vi "r3_sensor HDI placingerror.vi"() -> ()   [LabVIEW 2016]
uses:
  Classes/Controllers/Motion/Copy of Motion Folder/Motion.lvclass
  Classes/Controllers/Camera/Copy of Controller Folder/Controller.lvclass
panel:
  out "HDI center position from all time":dbl[][][](array[numeric])
  out "HDI-sensor deviation from all time":dbl[][][](array[numeric])
  out "HDI center position":dbl[][](array[numeric]) format="%#_8g"
  out "HDI bottom right":dbl[][](array[numeric]) format="%#_8g"
  out "HDI bottom left":dbl[][](array[numeric]) format="%#_8g"
  out "HDI top left":dbl[][](array[numeric]) format="%#_8g"
  in  "Default HDI A size":dbl[](array[numeric])=[24.3, 129.2, 78.448, 0.0001904]
  in  "Default HDI B size":dbl[](array[numeric])=[24.3, 101.2, 78.448, 0.0001904]
  in  "default HDI B top letf cross mark":dbl[](array[numeric])=[292.30913, 988.82841, 78.95, 0.00019035373]
  in  "default HDI A top left croos mark":dbl[](array[numeric])=[292.36164, 1091.0109, 78.95, 0.00019104402]
  out "measure times of HDI":dbl
  in  "Default sensor A size":dbl[](array[numeric])=[22.0, 129.5, 78.448, 0.0001904]
  in  "measure HDI position":bool
  in  "south - bottom right":bool
  in  "south - bottom left":bool
  in  "south - upper left":bool
  in  "north - bottom right":bool
  in  "north - bottom left":bool
  in  "north - upper left":bool
  out "HDI - sensor deviation on time":dbl[][](array[numeric]) format="%#_8g"
  out "HDI center position on time":dbl[][](array[numeric]) format="%#_8g"
  in  "default sensor A top left croos mark":dbl[](array[numeric])=[293.11276, 1090.4659, 78.600001, 0.00019004214]
  in  "test":bool
  in  "how much sensors":i32=2
  out "sensor bottom right":dbl[][](array[numeric]) format="%#_8g"
  out "sensor bottom left":dbl[][](array[numeric]) format="%#_8g"
  out "sensor top left":dbl[][](array[numeric]) format="%#_8g"
  out "sensor center position":dbl[][](array[numeric]) format="%#_8g"
  in  "default sensor B top letf cross mark":dbl[](array[numeric])=[293.05065, 988.27536, 78.609997, 0.00018966104]
  in  "Default sensor B size":dbl[](array[numeric])=[22.0, 101.5, 78.448, 0.0001904]
  out "measure times of sensor":dbl
  in  "Parking position":dbl[](array[numeric])=[625.0, 625.0, 0.0, 0.01]
  in  "measure sensor position":bool
  in  "calculate":bool
  in  "go to park":bool
  in  "stop":bool
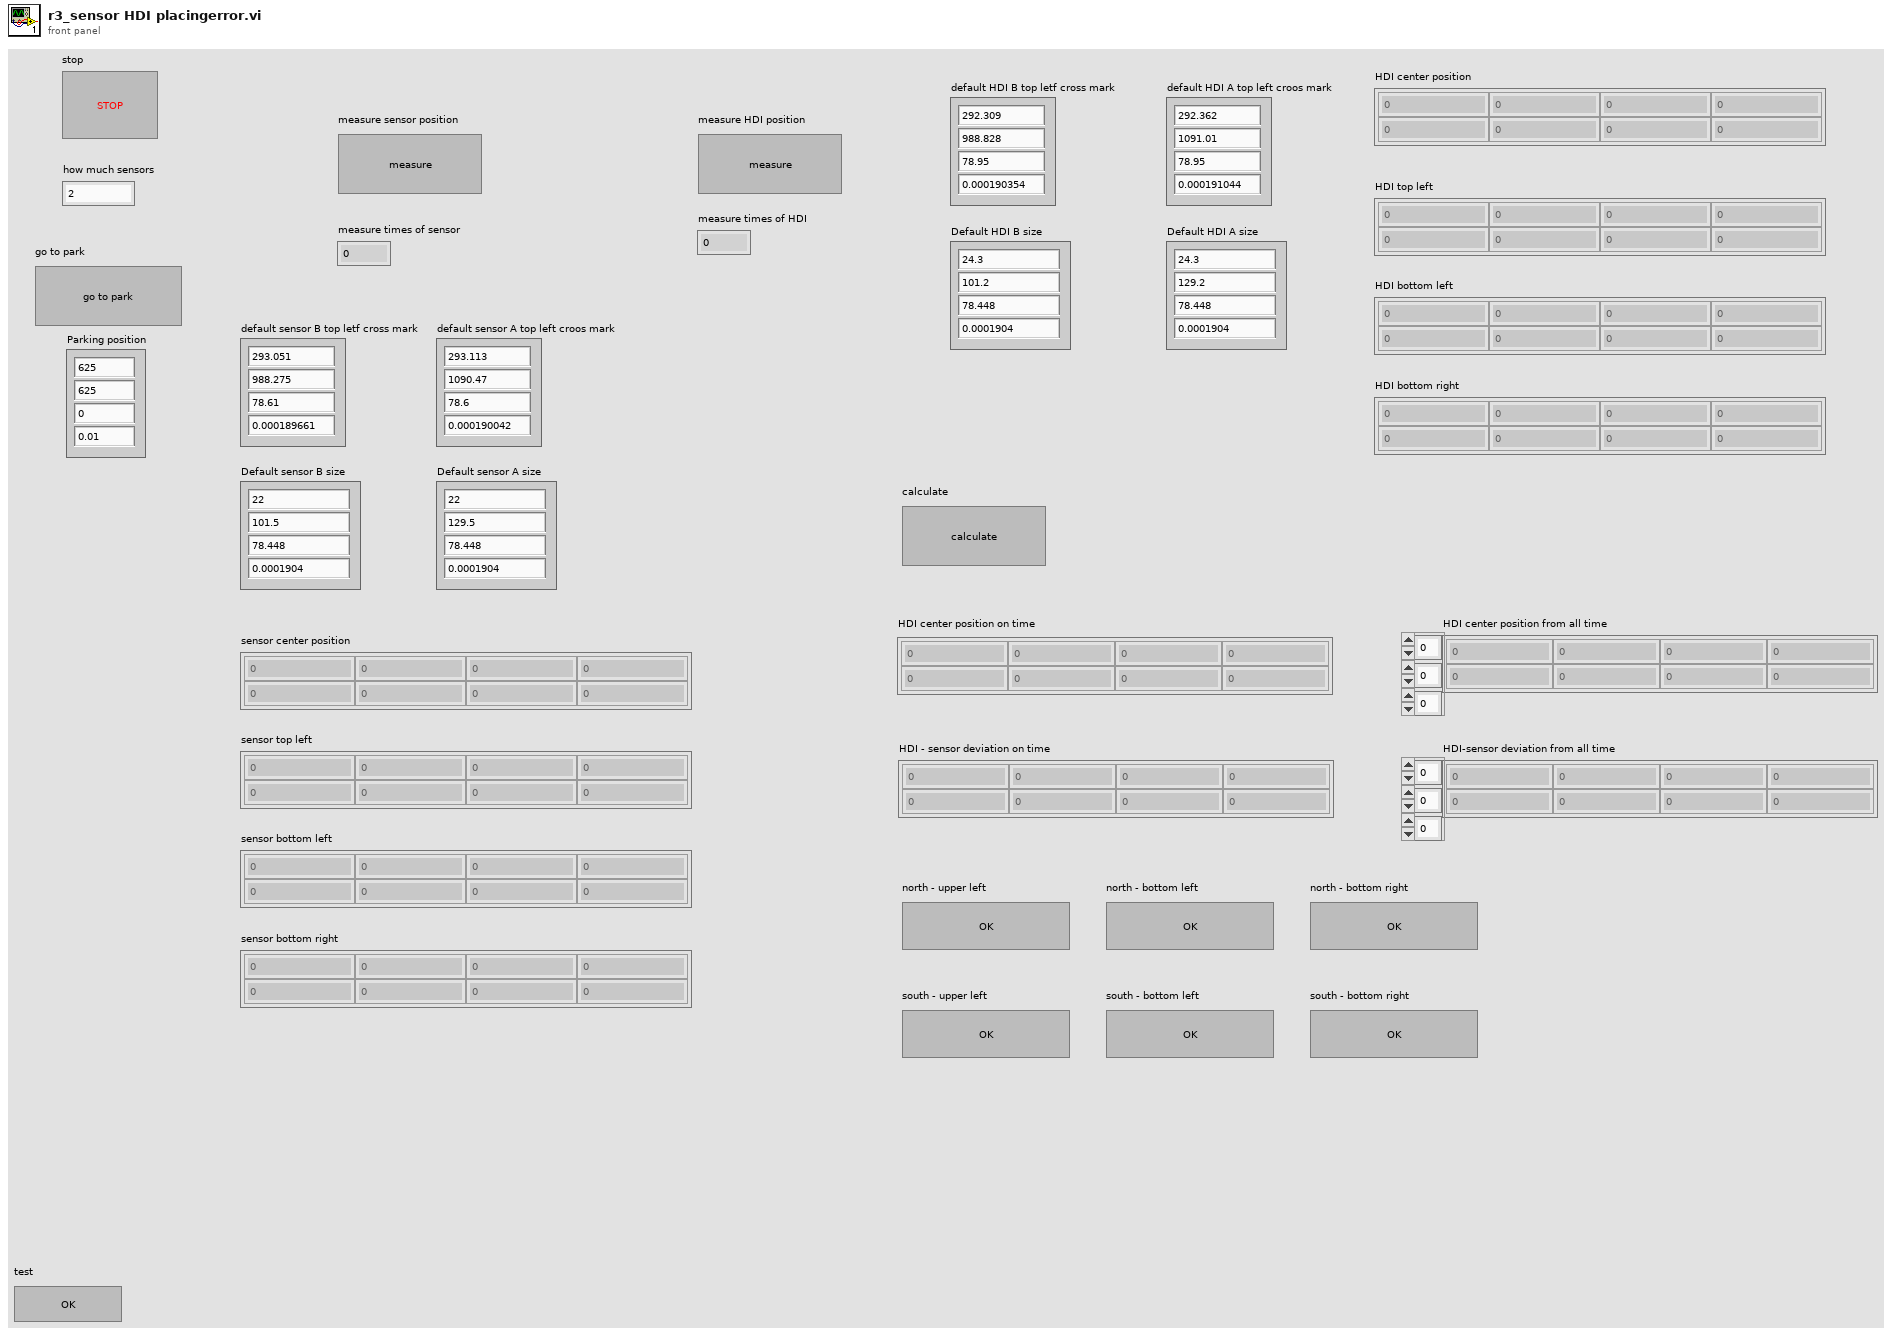
[diagram p1: front panel]
types:
  T1 = typedef "Controller.lvclass/Controllers.ctl" = cluster{"Copy of Motion.lvclass":refnum<class "Motion.lvclass">, "Copy of I-O.lvclass":refnum<class "I-O.lvclass">, "Copy of Dispenser.lvclass":refnum<class "Dispenser.lvclass">}
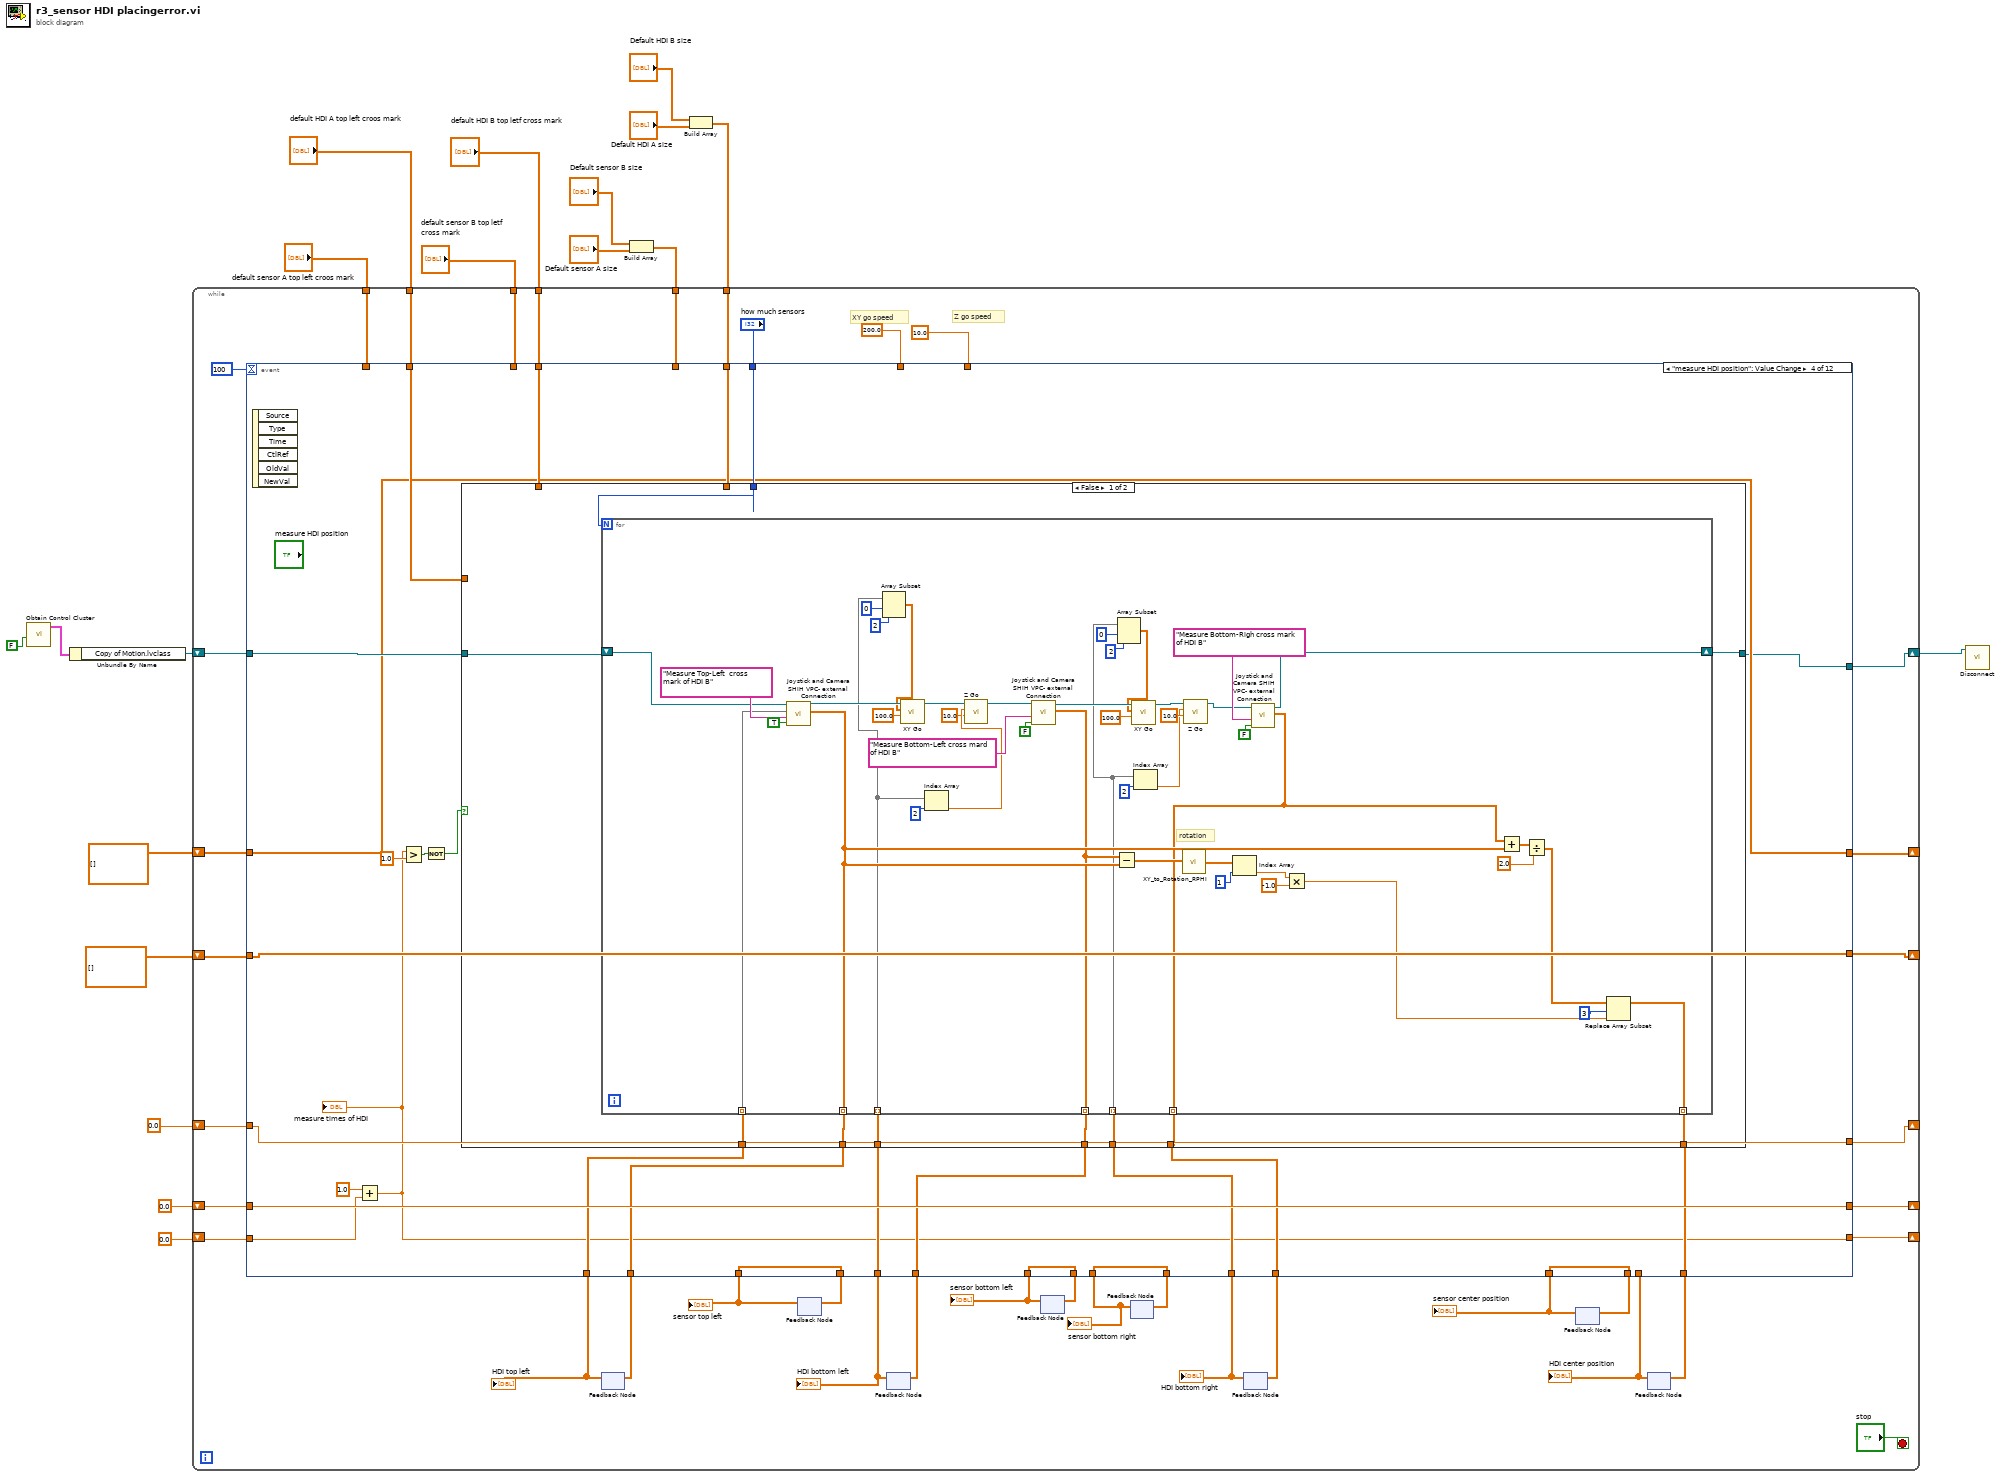
[diagram p0: block diagram]
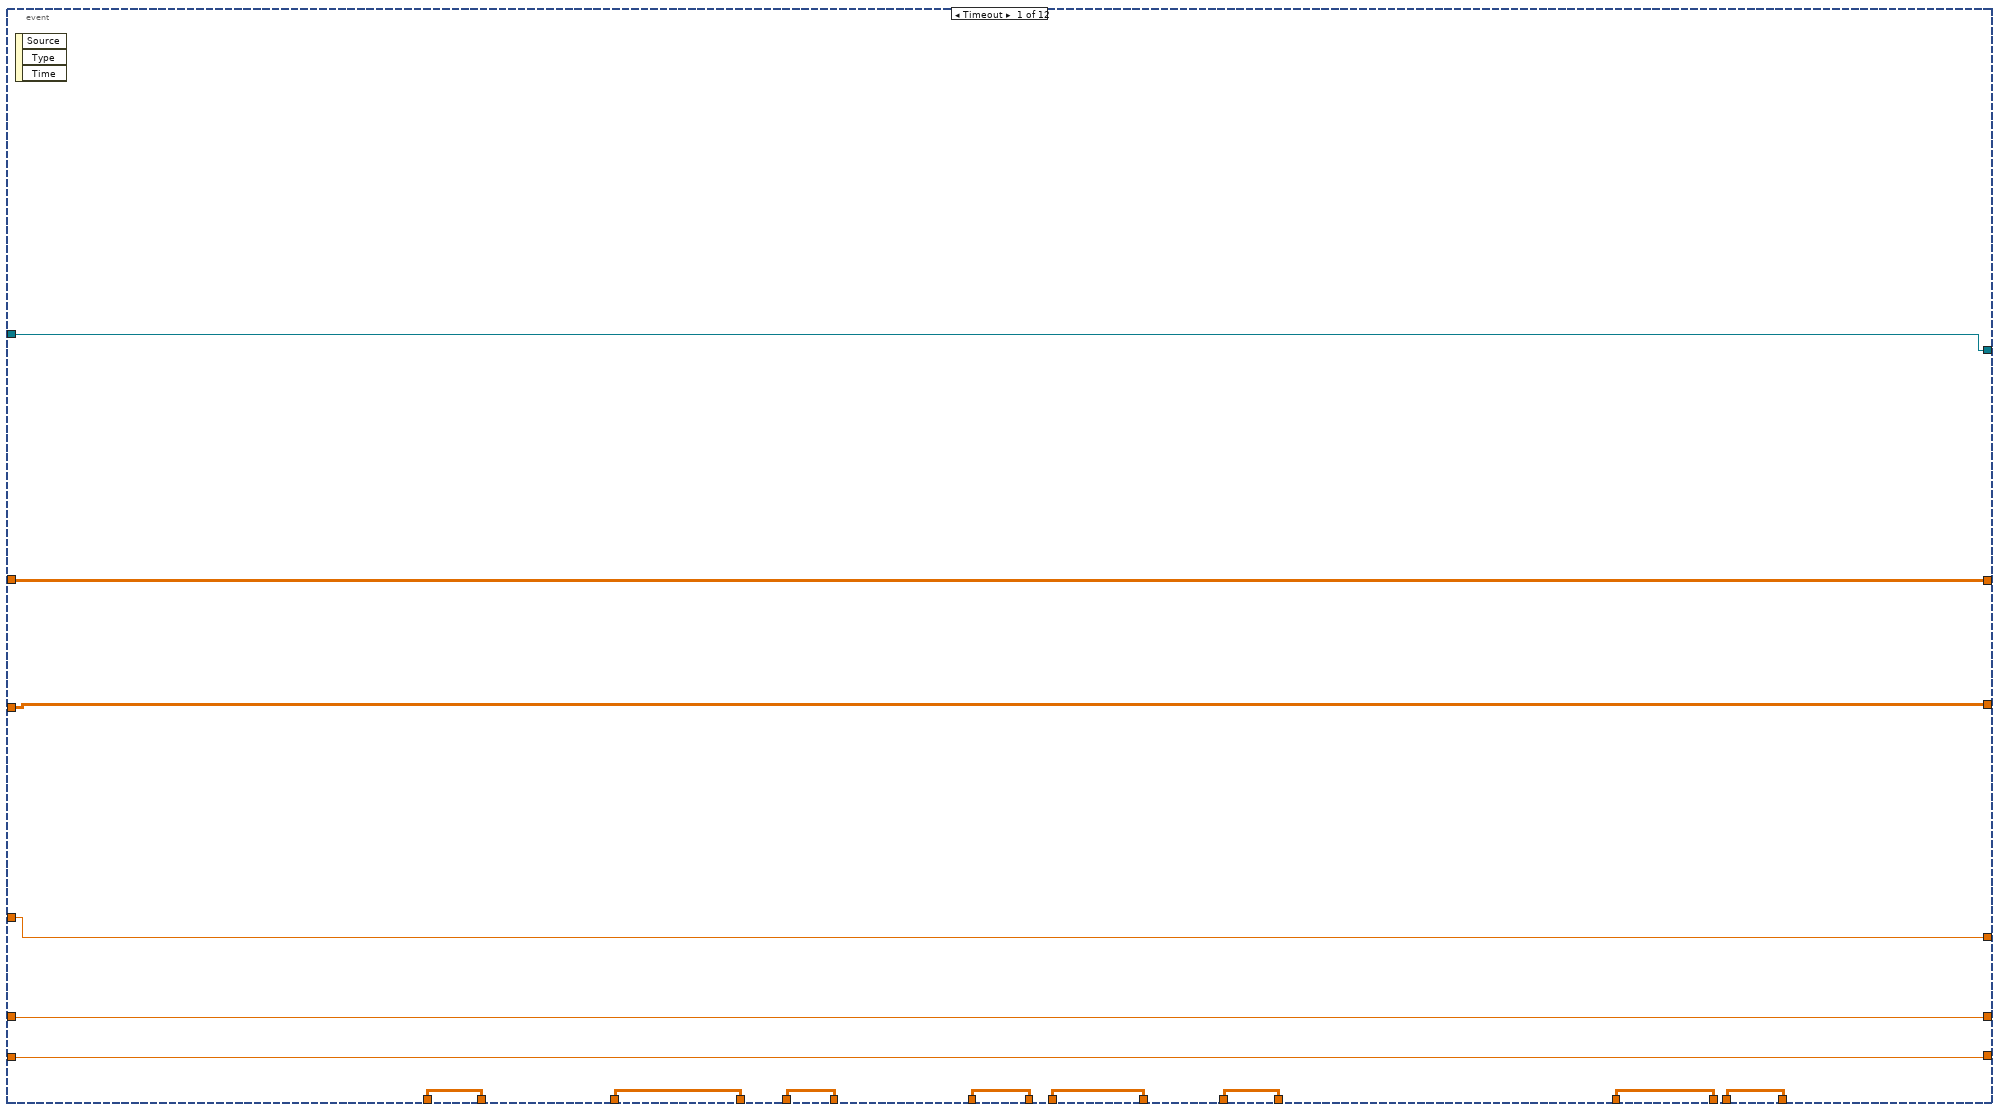
[diagram p2: hidden frame]
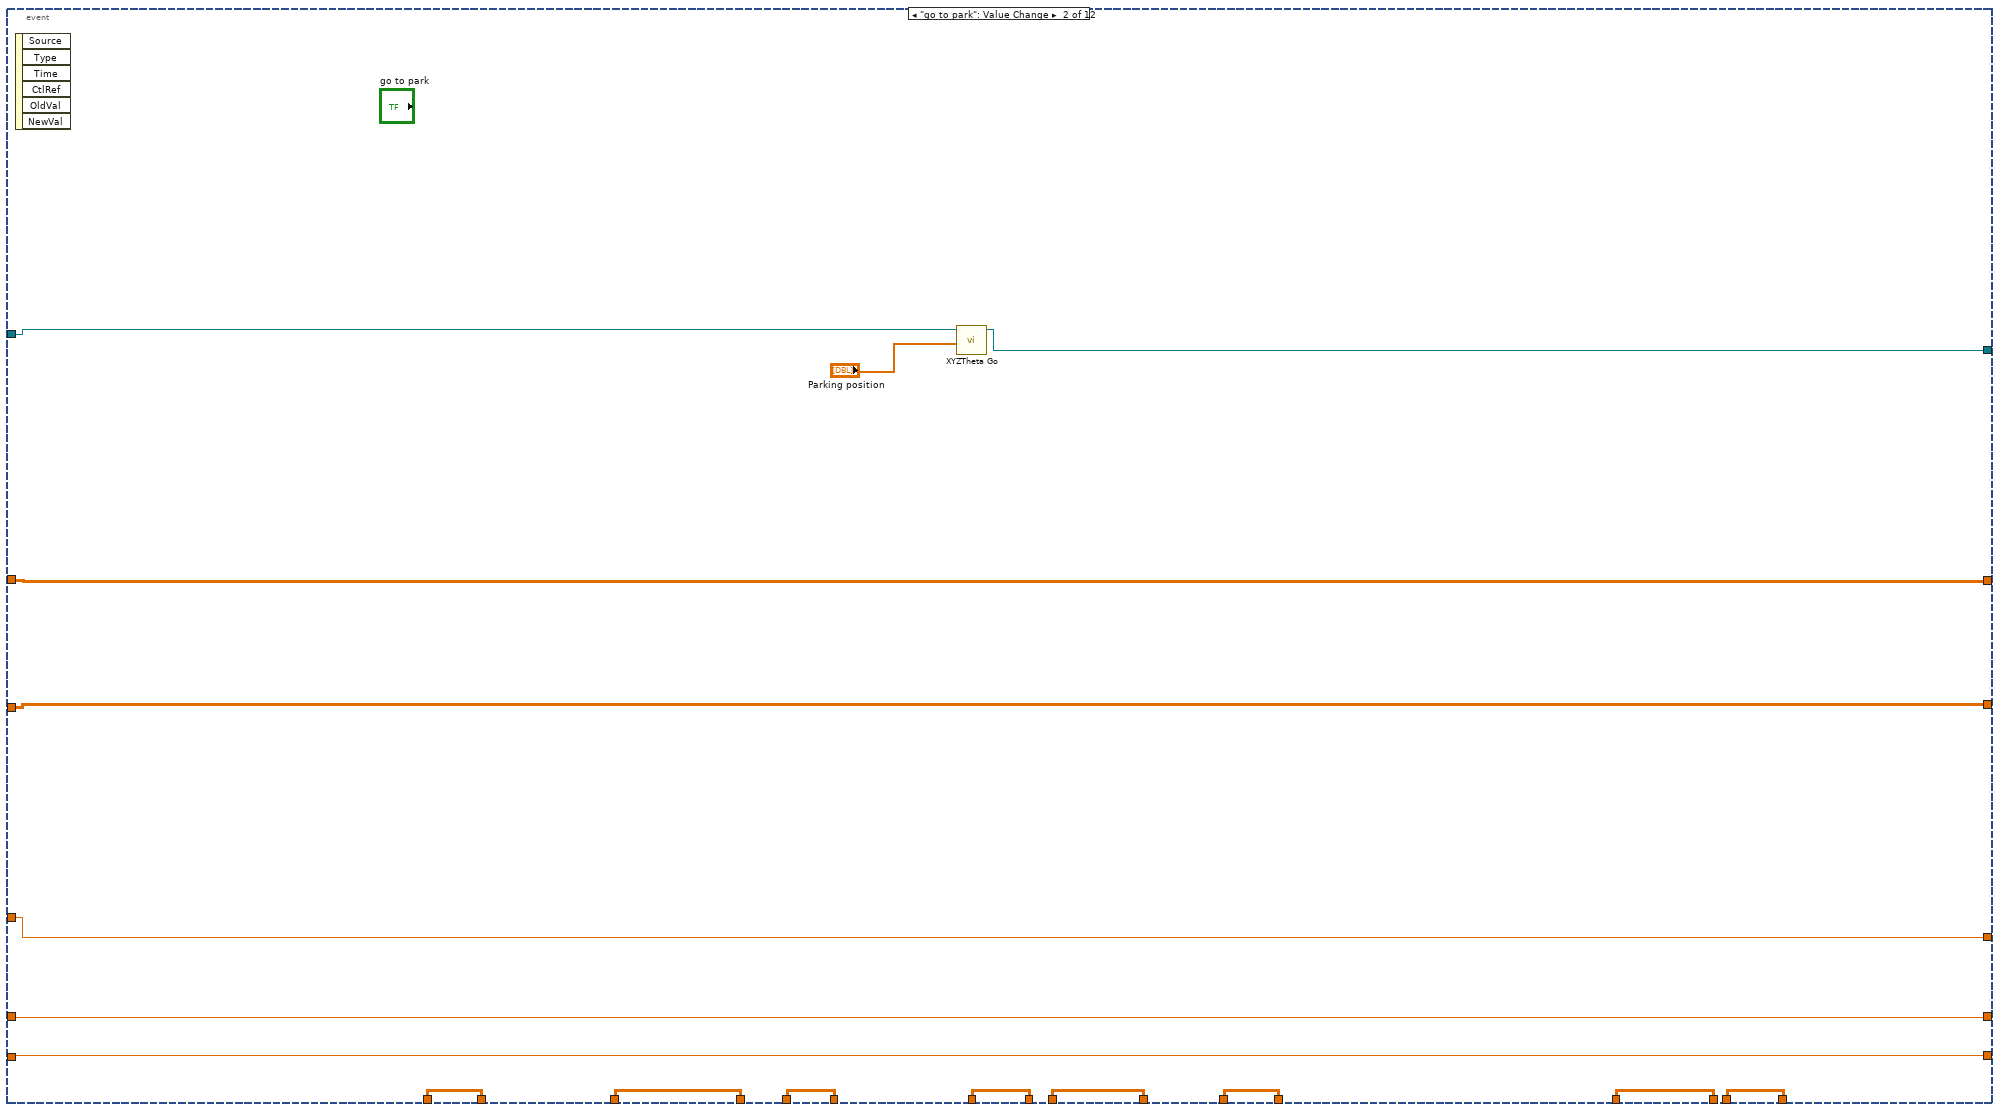
[diagram p3: hidden frame]
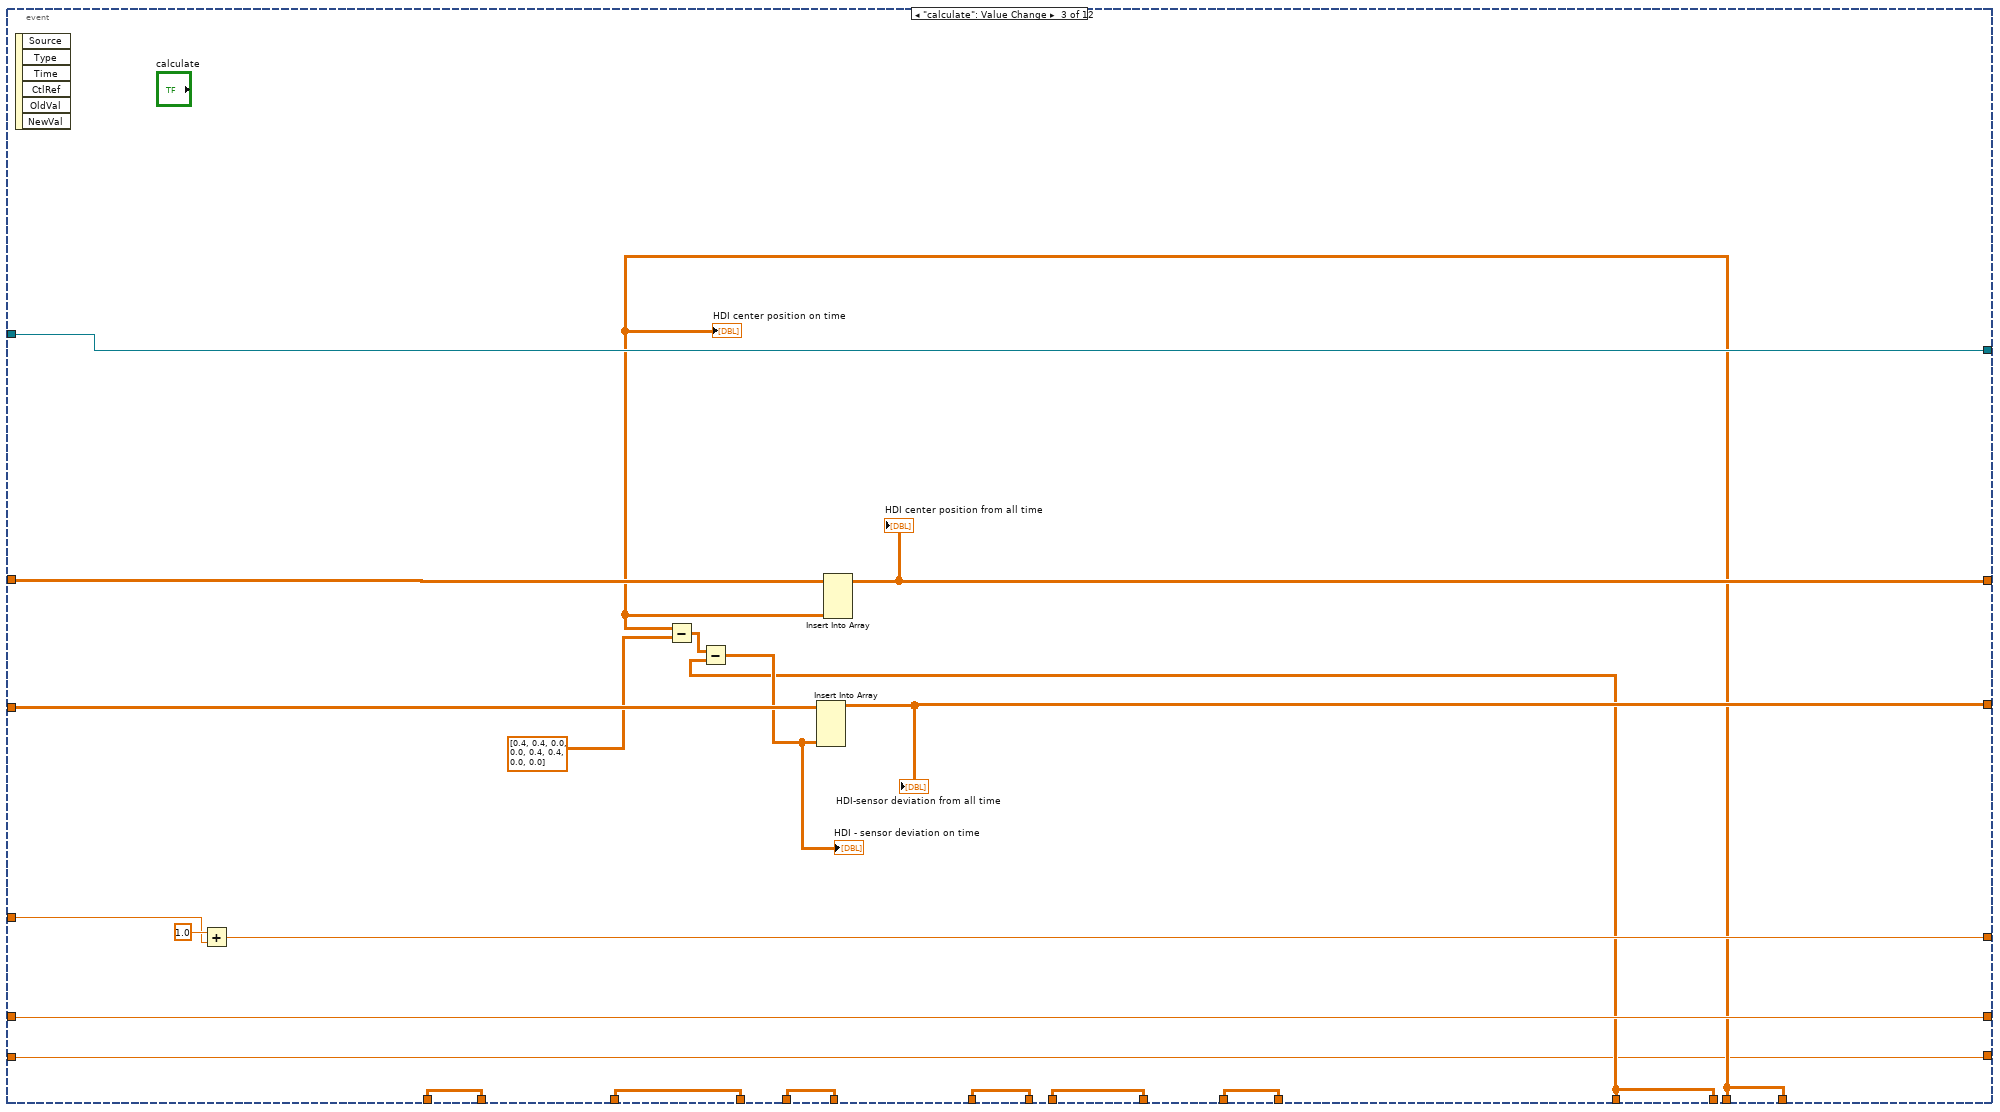
[diagram p4: hidden frame]
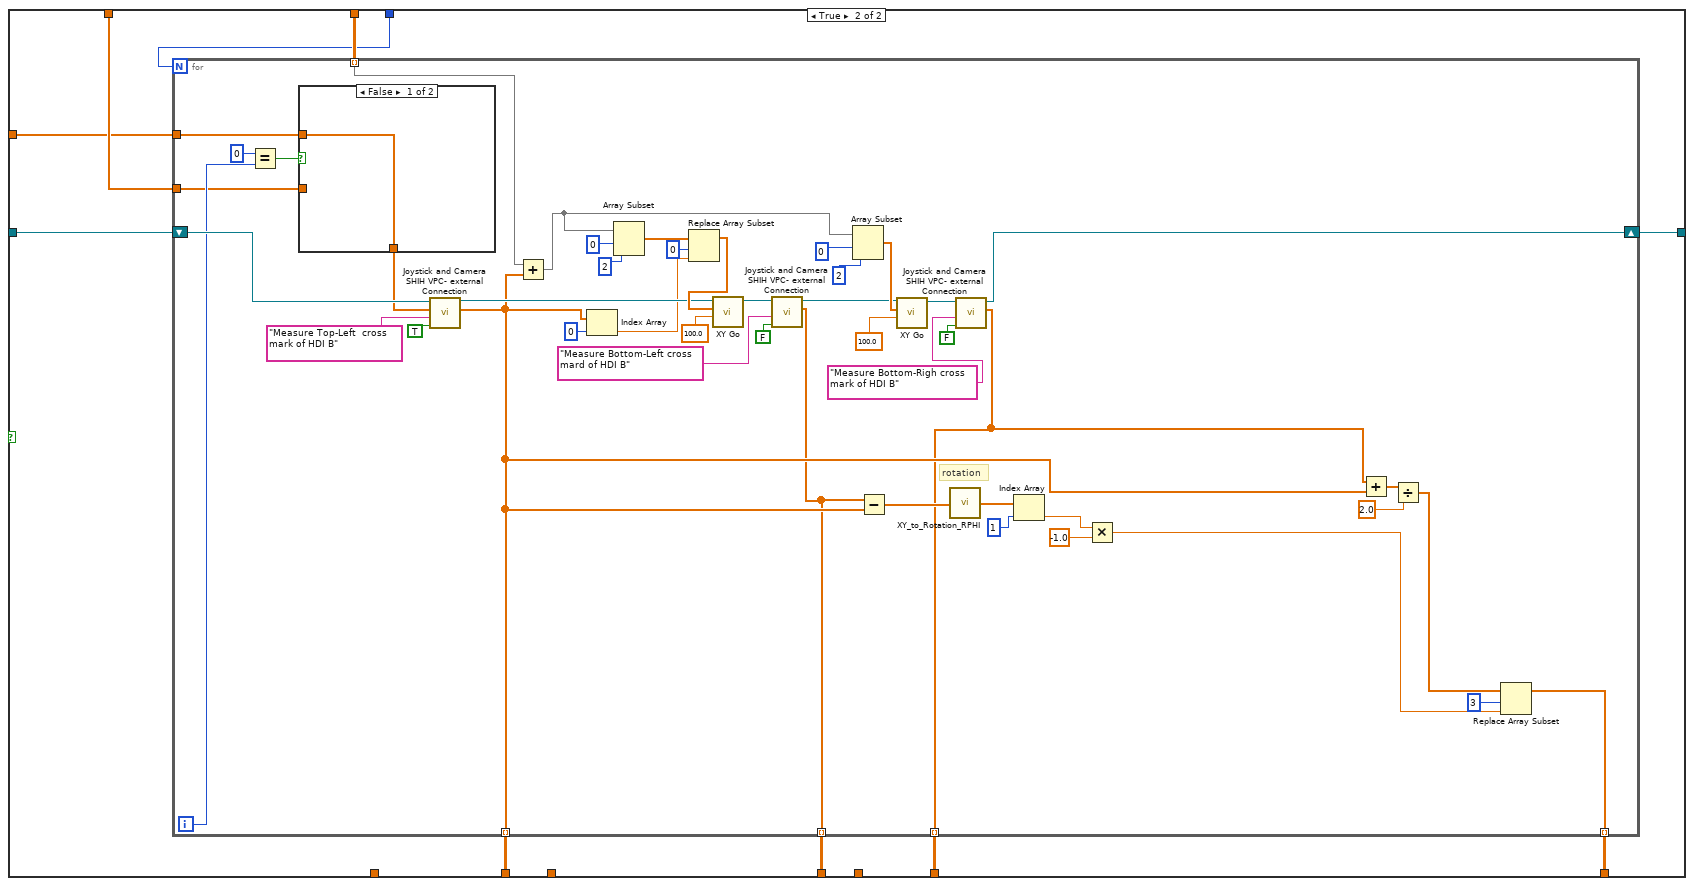
[diagram p5: hidden frame]
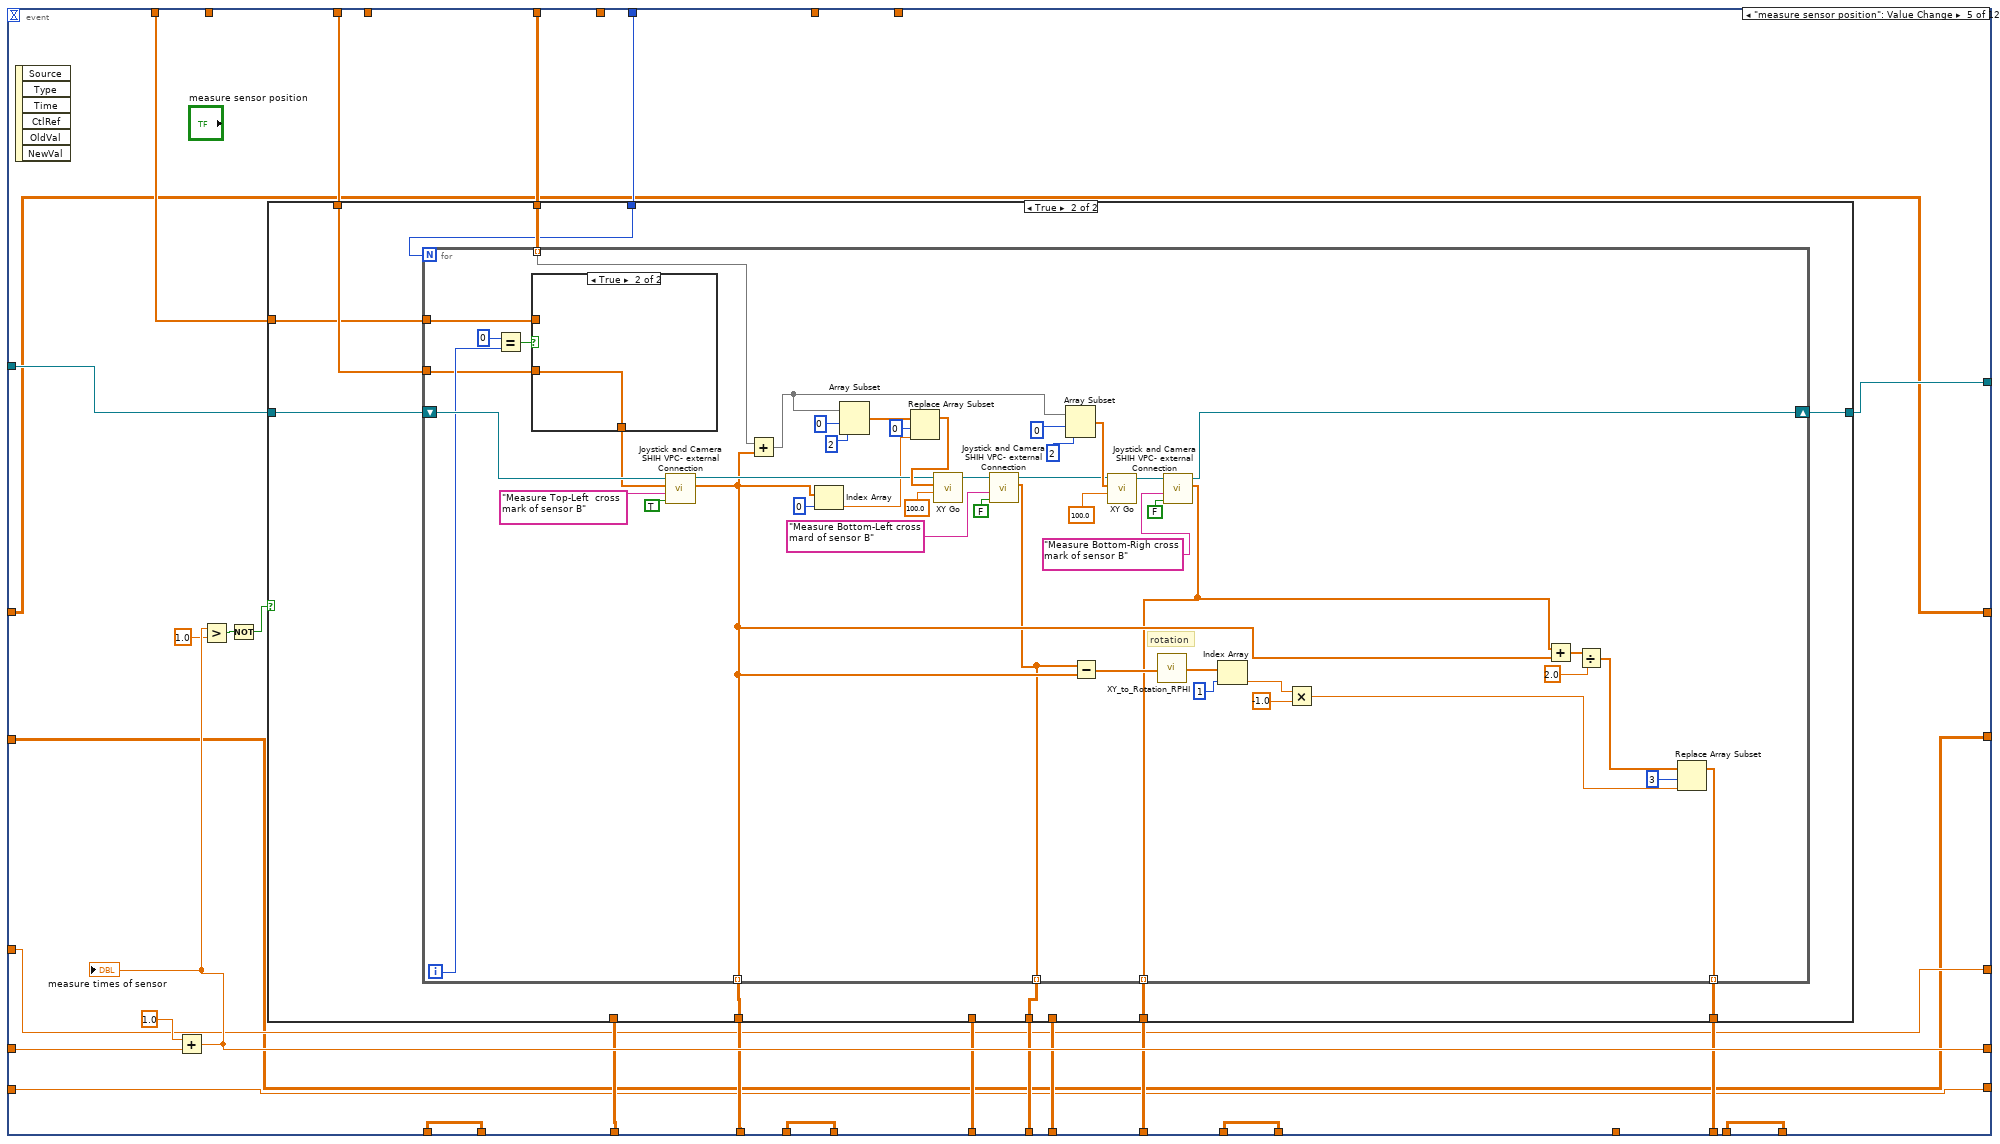
[diagram p7: hidden frame]
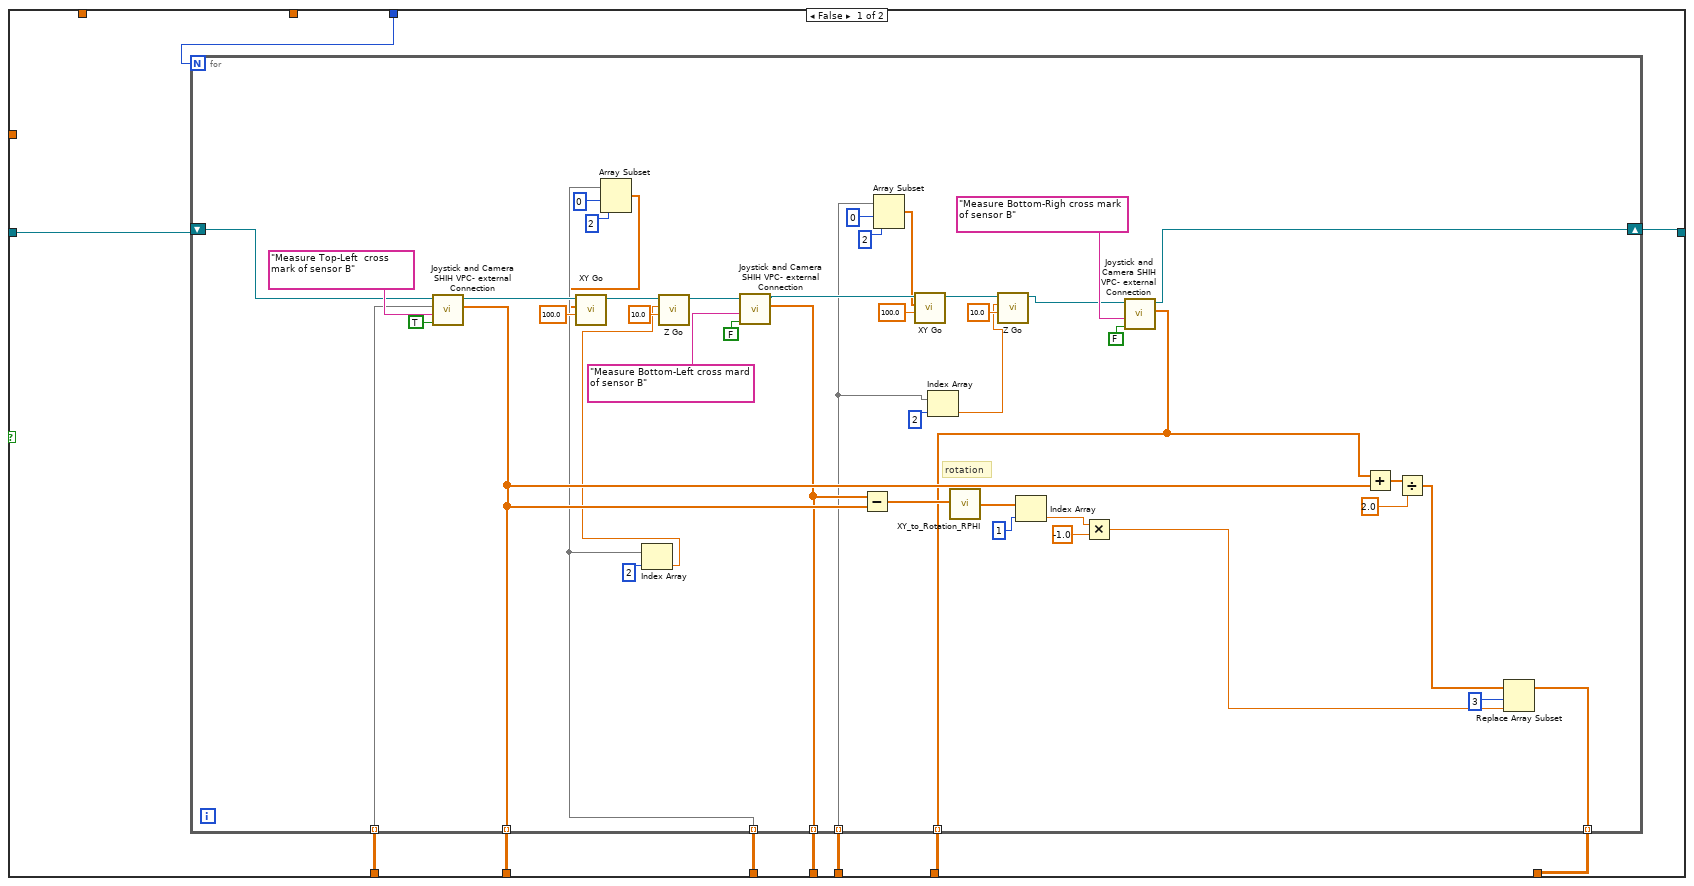
[diagram p8: hidden frame]
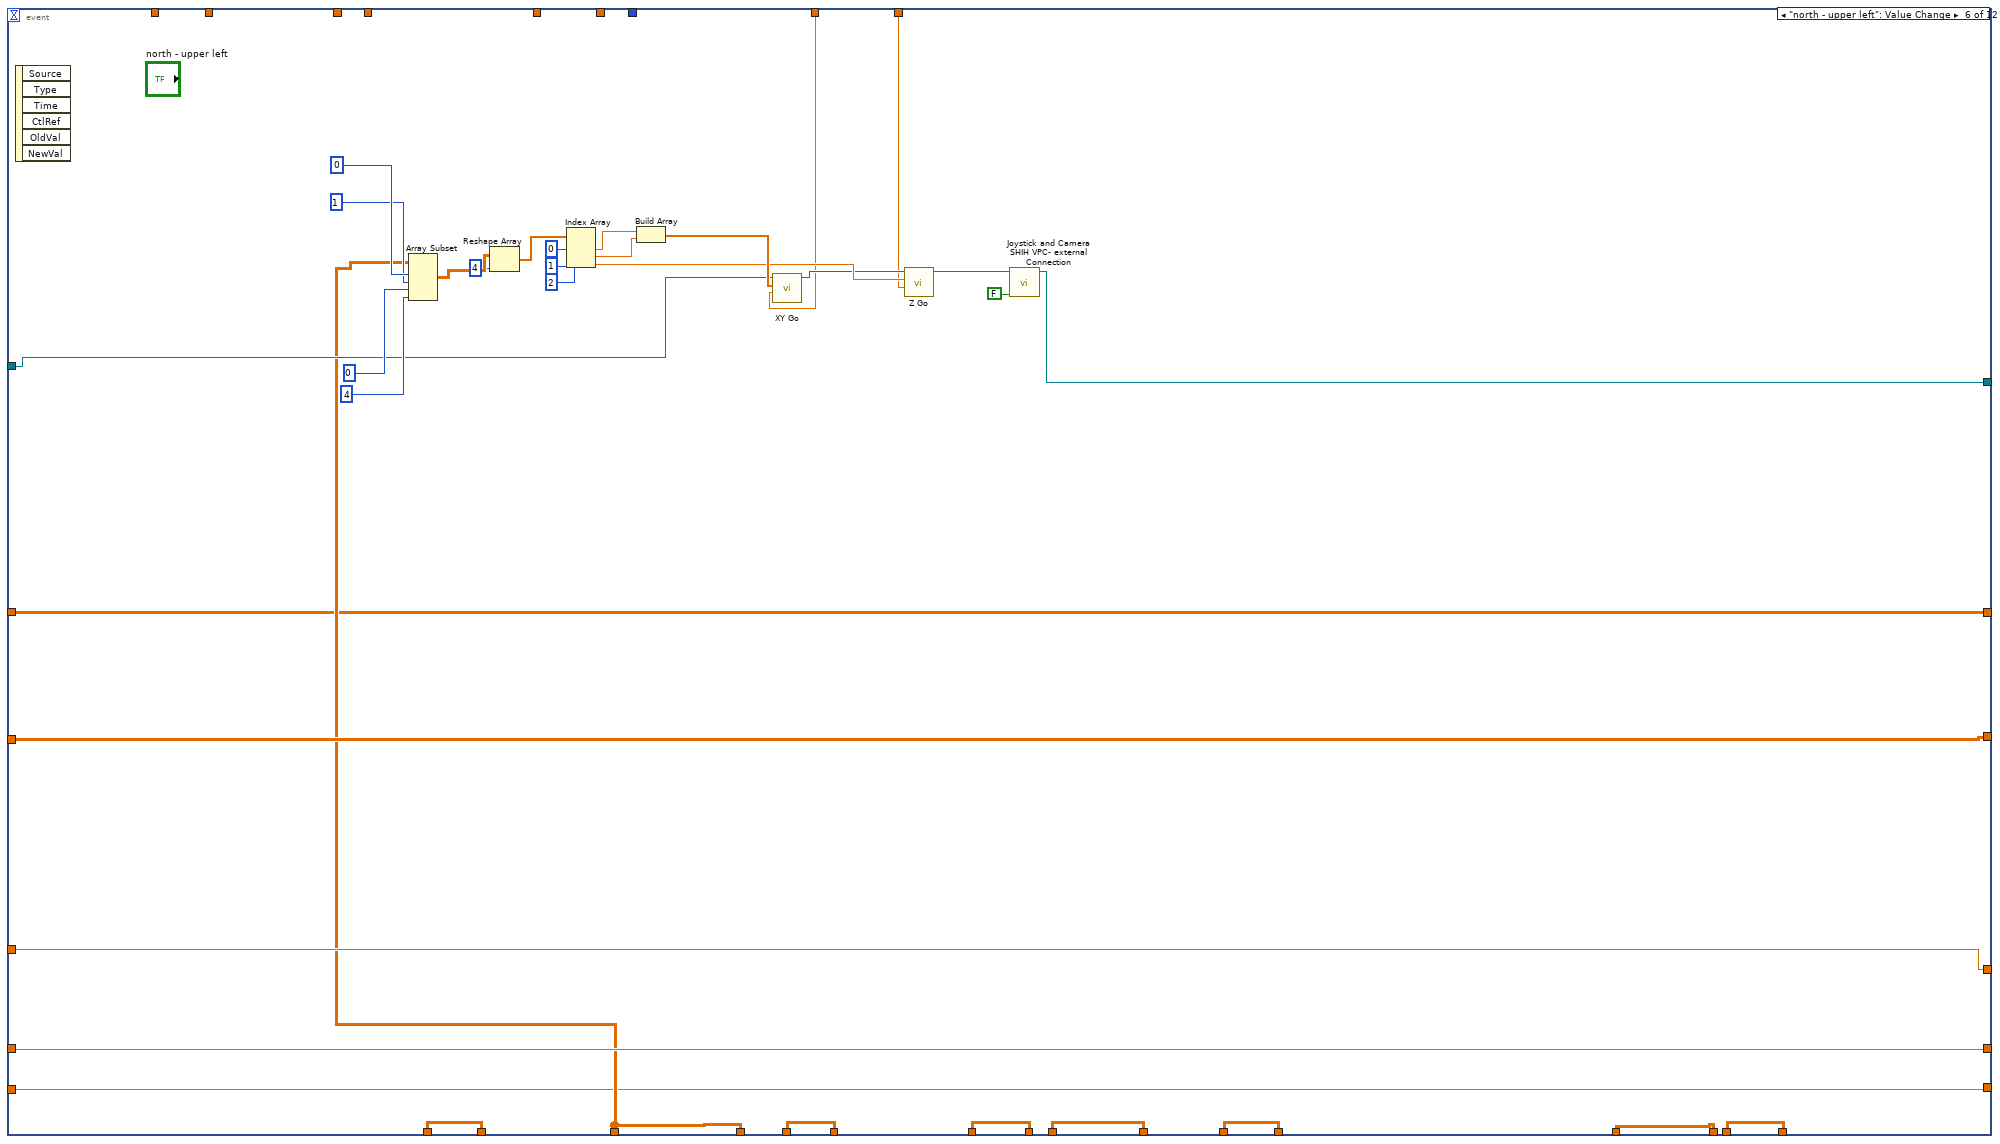
[diagram p10: hidden frame]
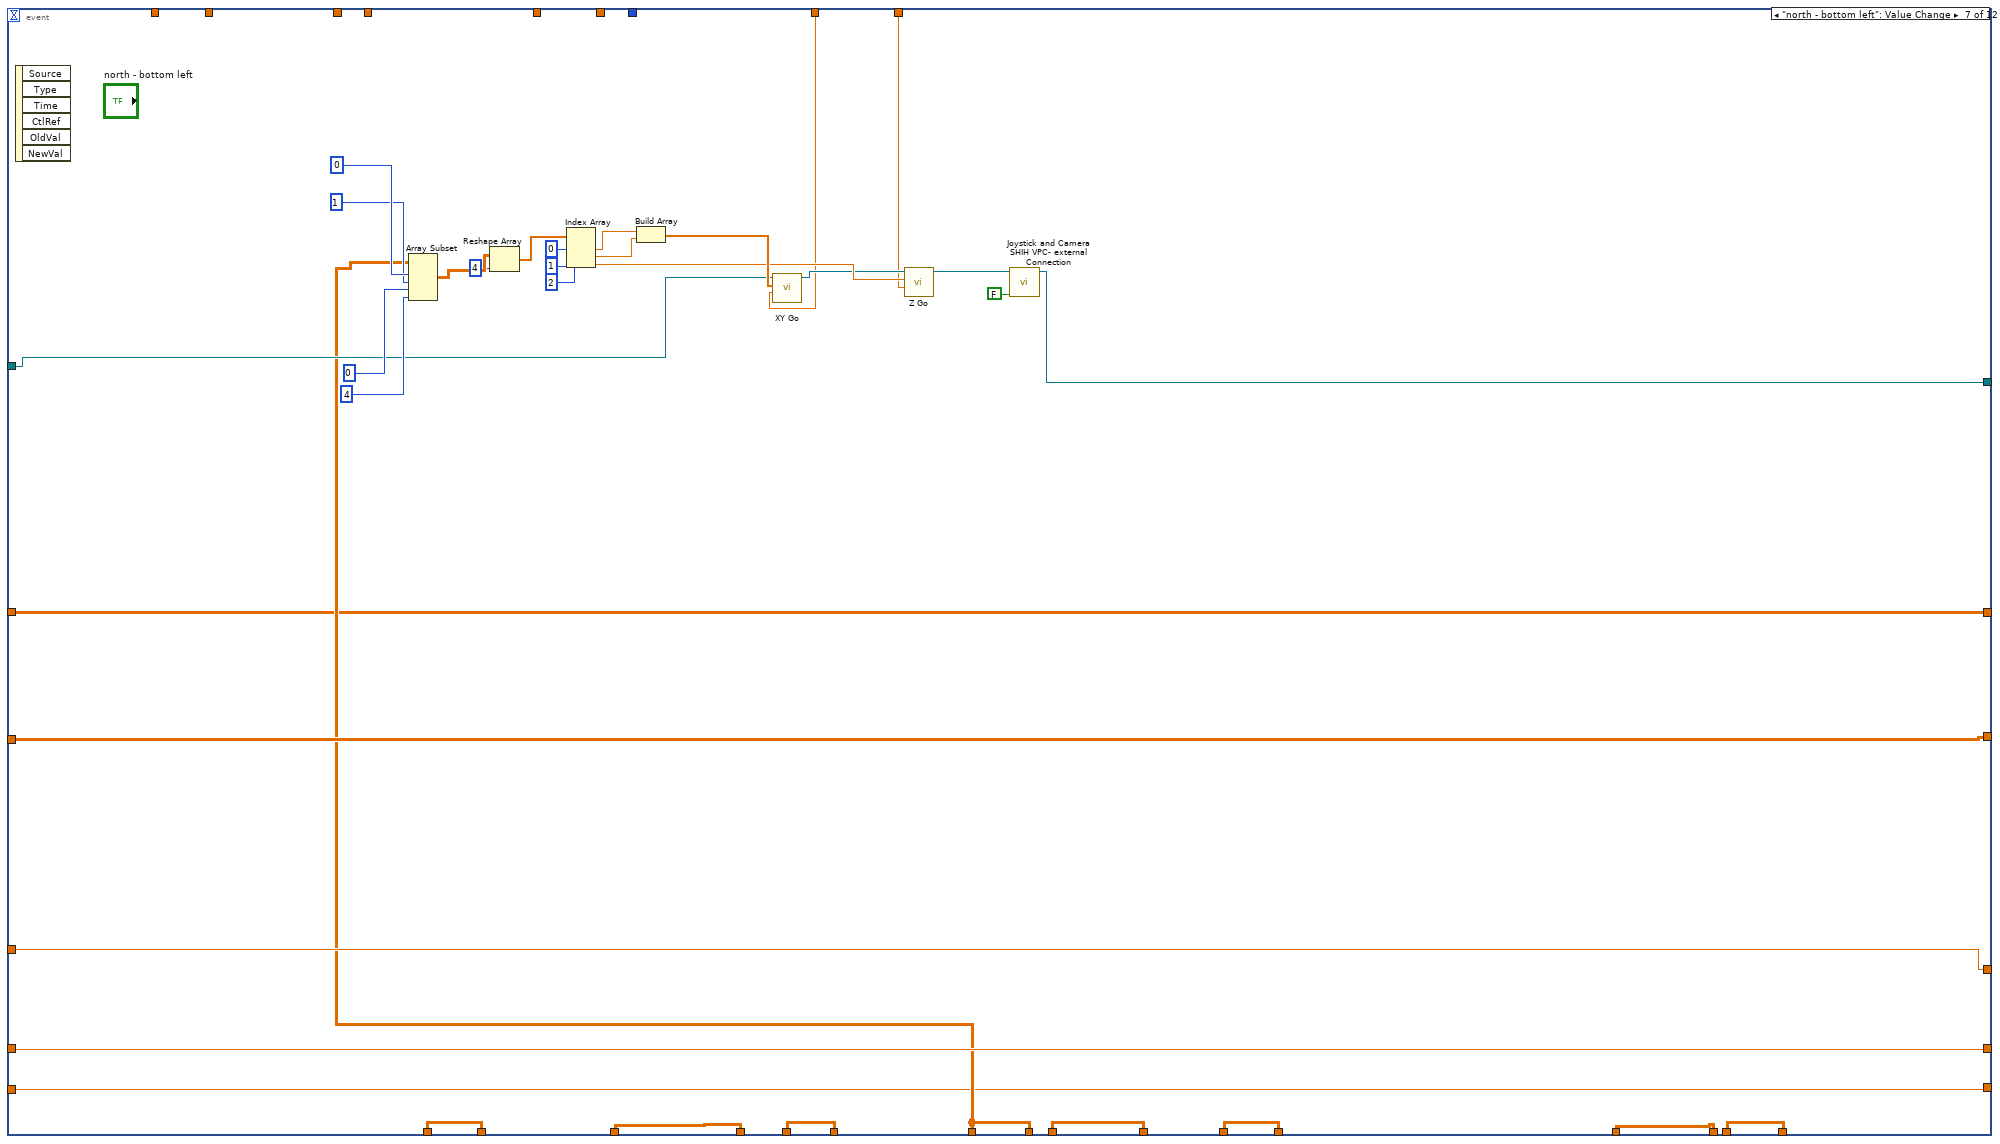
[diagram p11: hidden frame]
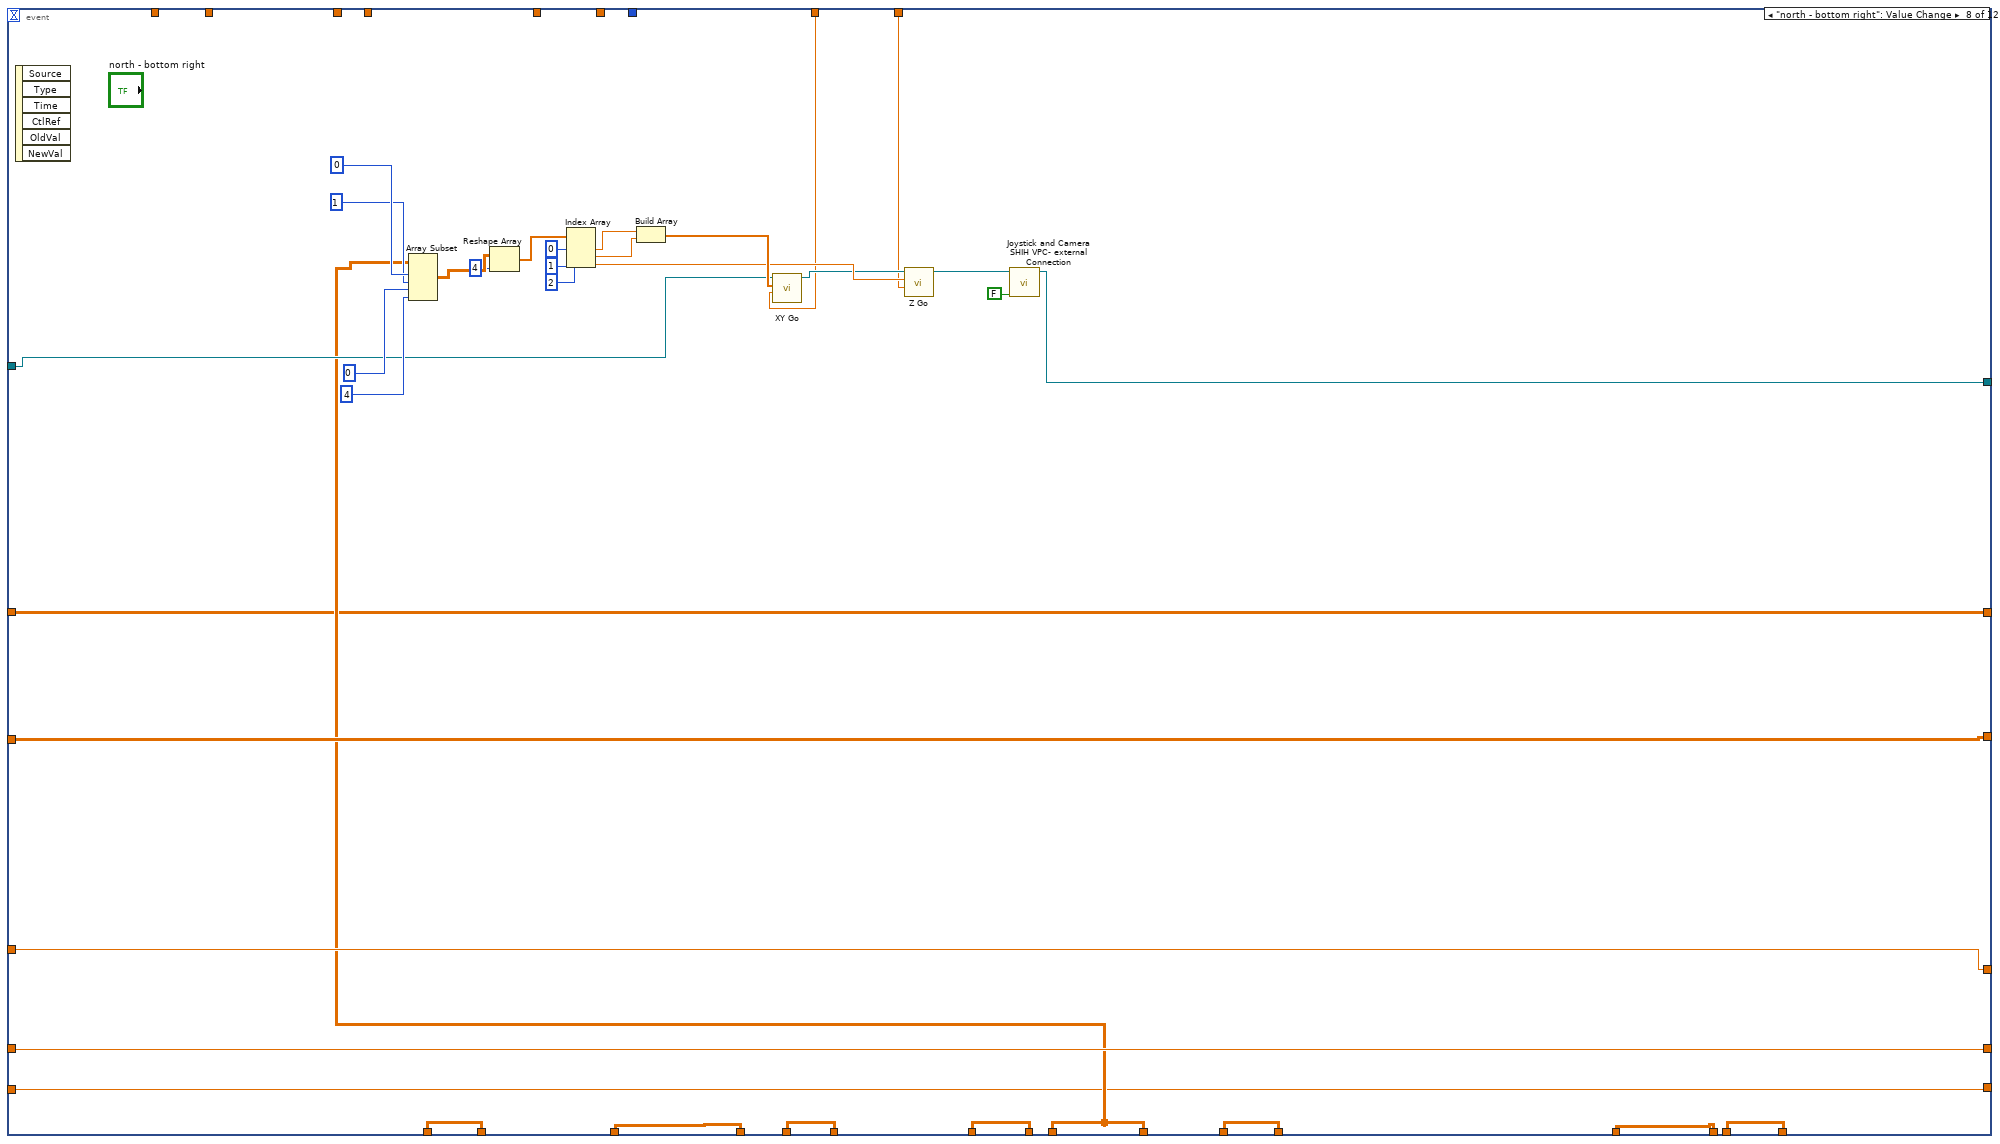
[diagram p12: hidden frame]
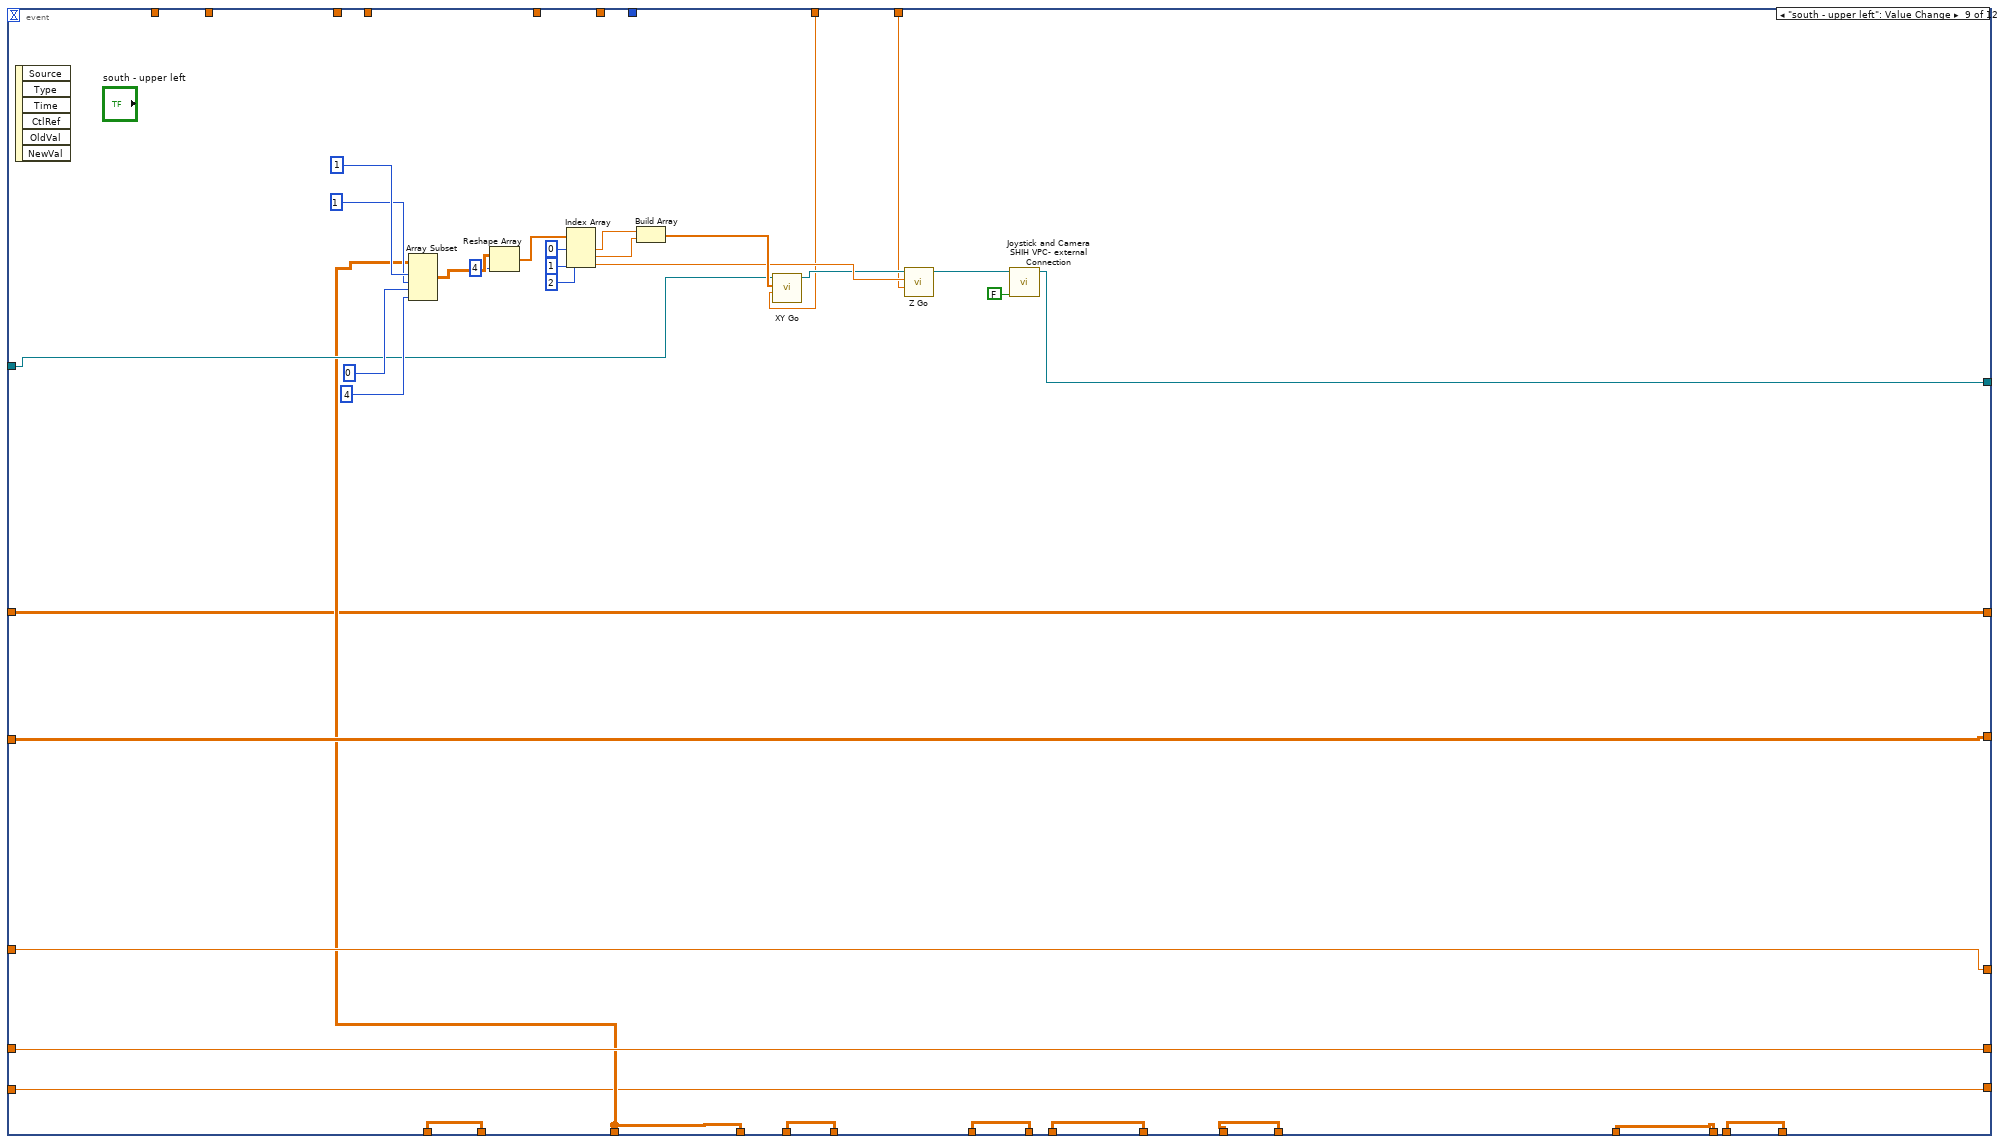
[diagram p13: hidden frame]
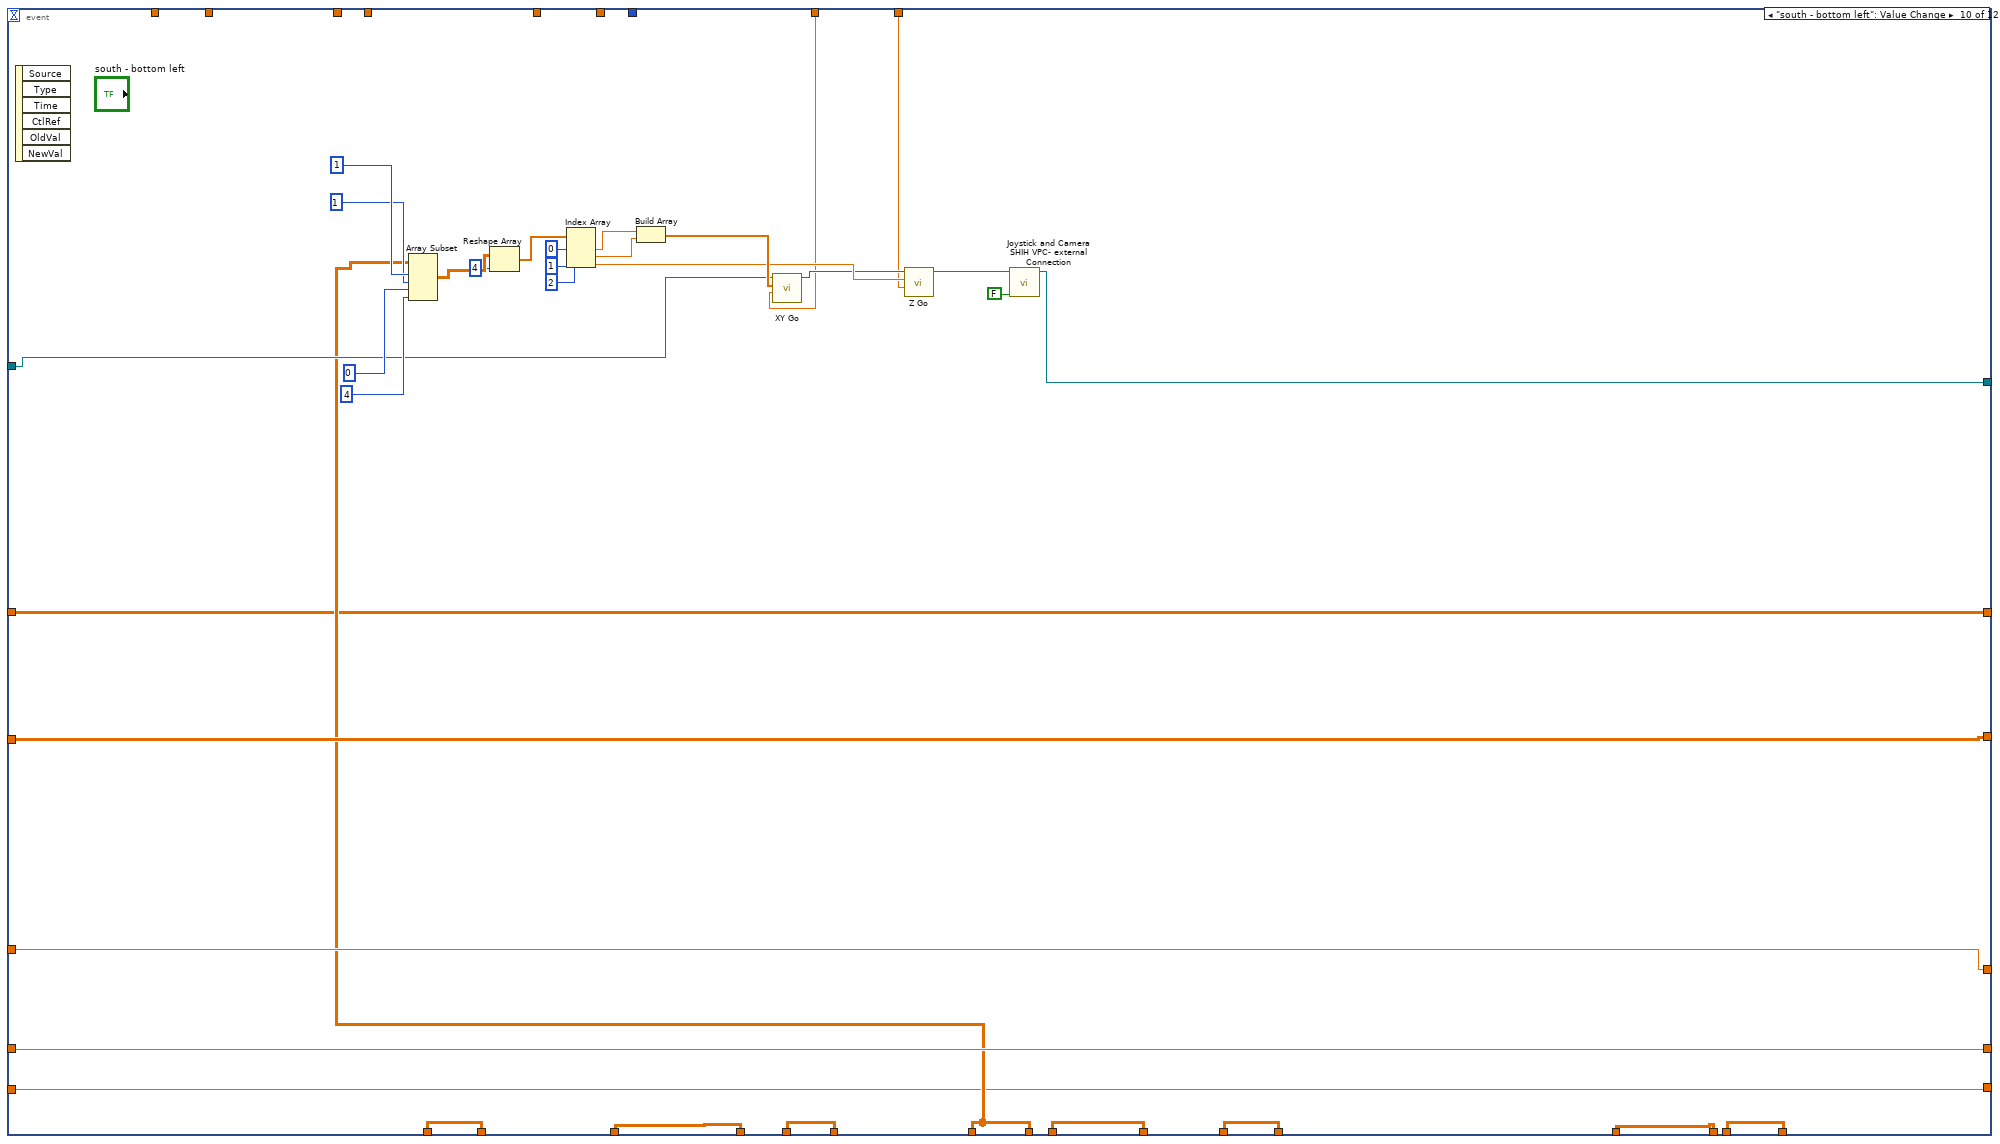
[diagram p14: hidden frame]
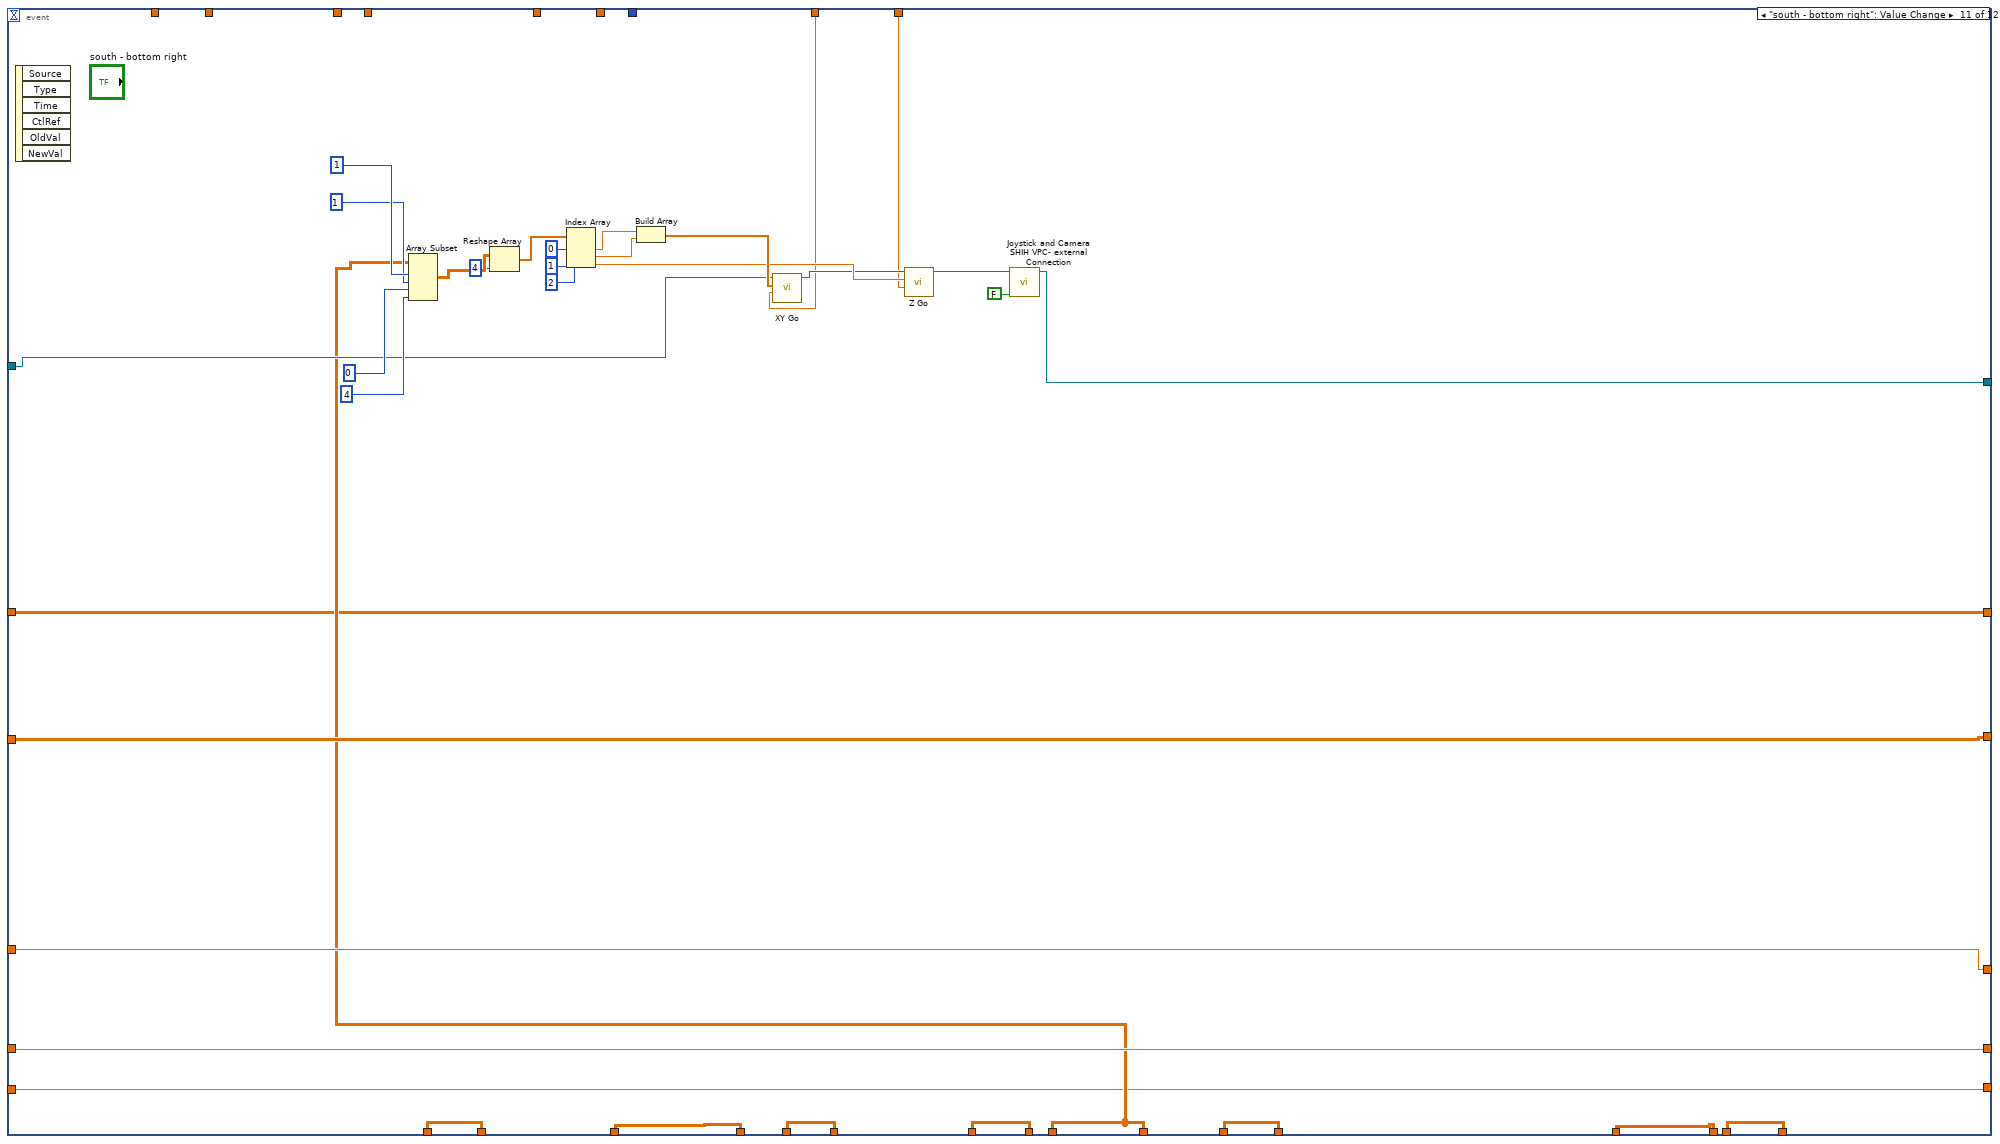
[diagram p15: hidden frame]
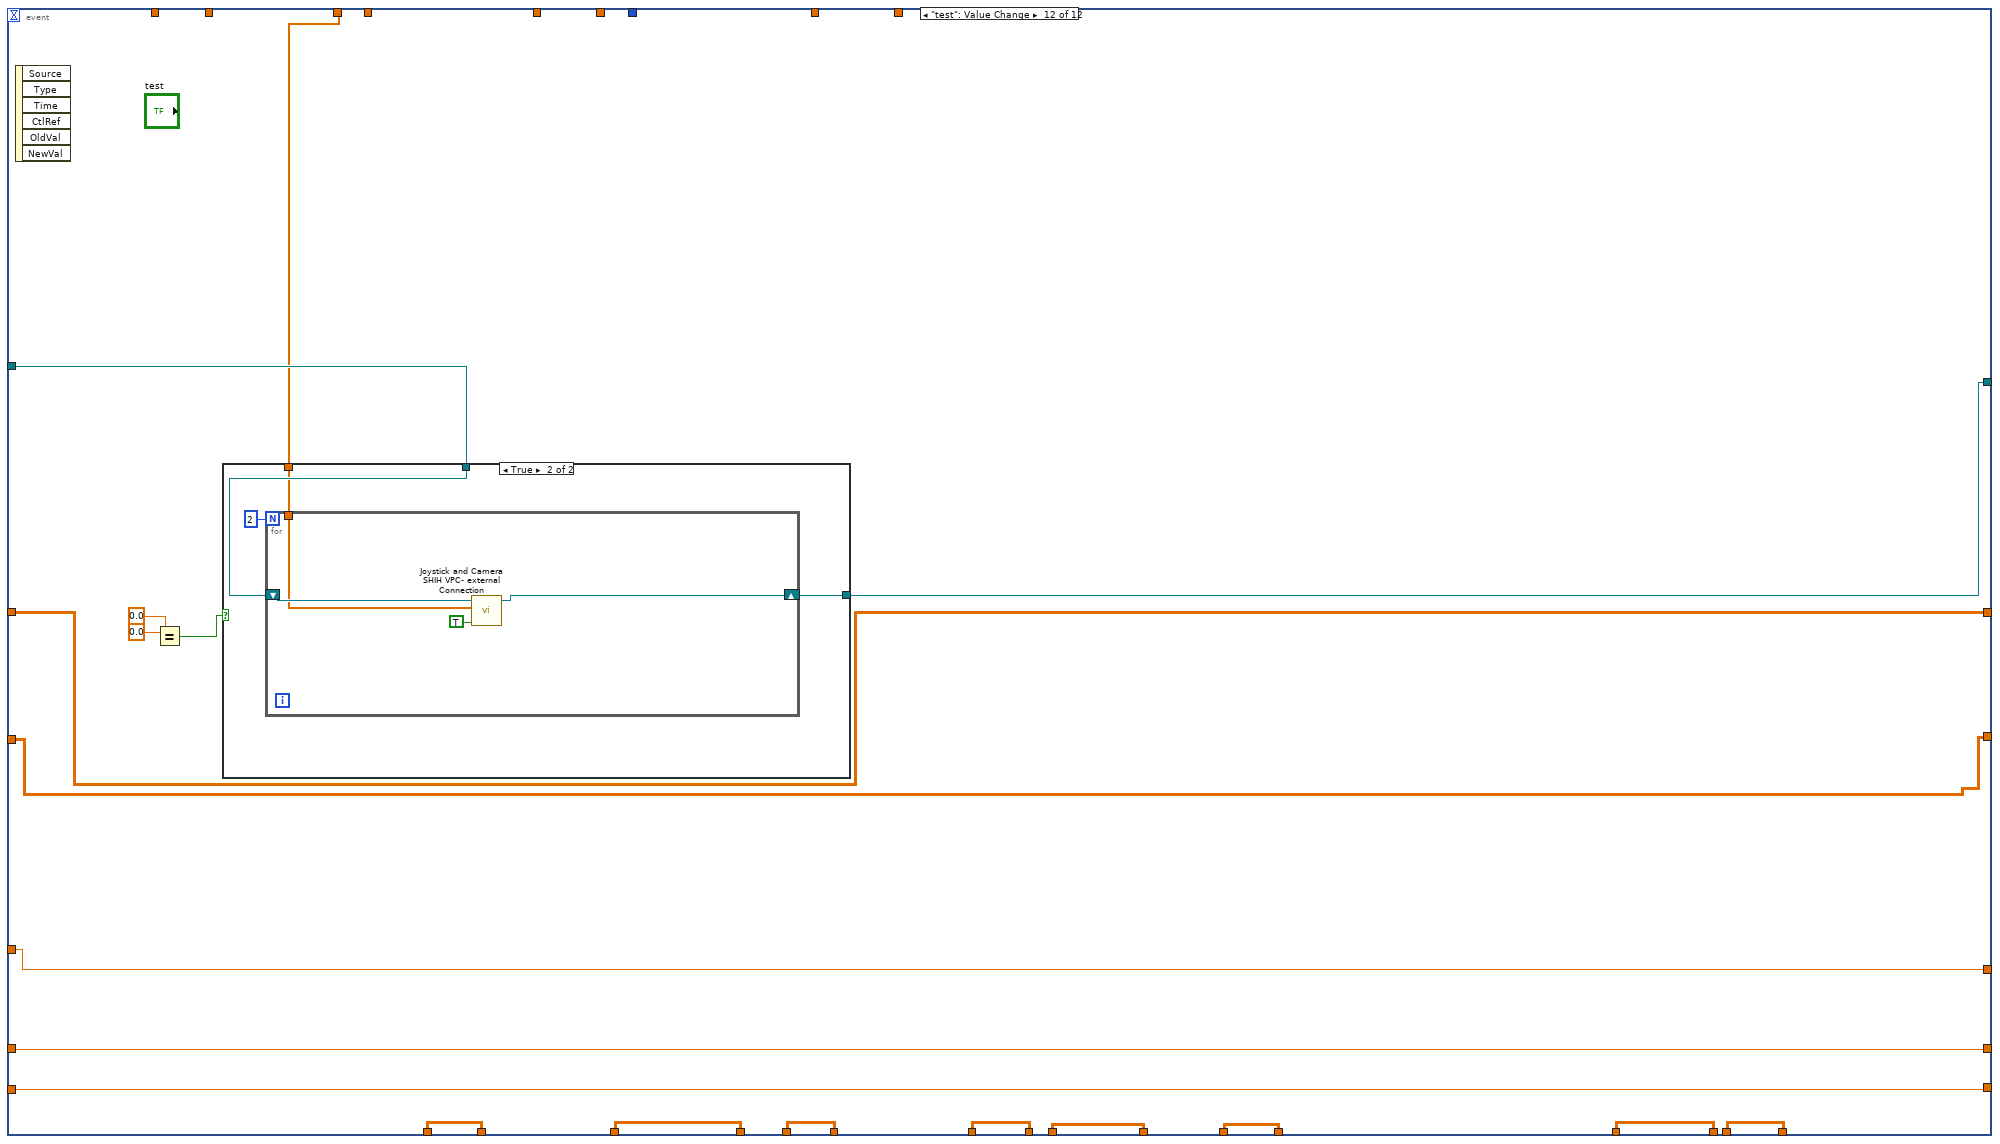
[diagram p16: hidden frame]
diagram:
  n1 = call "Obtain Control Cluster.vi"("I/O"=FALSE) -> ("Control Out"=w19:T1)  [unwired: 10 in]
  n2 = Unbundle By Name(w19) -> ("Copy of Motion.lvclass"=w17:refnum<class "Motion.lvclass">)
  n3 = Build Array("Default sensor B size", "Default sensor A size") -> (w8:dbl[][])
  n4 = Build Array("Default HDI B size", "Default HDI A size") -> (w3:dbl[][])
  n5 = while {
    shift-right: [w55] -> w16
    shift-left: w17 -> [w56]
    shift-right: [w53] -> _
    shift-left: 0.0 -> [w54]
    tunnel: w8 -> [w52]
    tunnel: "default sensor B top letf cross mark" -> [w51]
    tunnel: "default sensor A top left croos mark" -> [w42]
    shift-right: [w39] -> _
    shift-left: 0.0 -> [w40]
    shift-right: [w37] -> _
    shift-left: dbl[][][] [] -> [w38]
    tunnel: "default HDI A top left croos mark" -> [w34]
    tunnel: "default HDI B top letf cross mark" -> [w33]
    tunnel: w3 -> [w32]
    shift-right: [w23] -> _
    shift-left: dbl[][][] [] -> [w22]
    shift-right: [w20] -> _
    shift-left: 0.0 -> [w21]
    stop <- "stop" stop-if-true
    # "Z go speed"
    # "XY go speed"
    n6 = feedback #1() -> (w26:dbl[][])  [unwired: 1 in]
    "HDI top left" <- w26
    n7 = feedback #2() -> (w48:dbl[][])  [unwired: 1 in]
    "sensor top left" <- w48
    n8 = feedback #3() -> (w28:dbl[][])  [unwired: 1 in]
    "HDI bottom left" <- w28
    n9 = feedback #4() -> (w45:dbl[][])  [unwired: 1 in]
    "sensor bottom left" <- w45
    n10 = feedback #5() -> (w44:dbl[][])  [unwired: 1 in]
    "sensor bottom right" <- w44
    n11 = feedback #6() -> (w30:dbl[][])  [unwired: 1 in]
    "HDI bottom right" <- w30
    n12 = feedback #7() -> (w41:dbl[][])  [unwired: 1 in]
    "sensor center position" <- w41
    n13 = feedback #8() -> (w24:dbl[][])  [unwired: 1 in]
    "HDI center position" <- w24
    n14 = event shown="[3] \"measure HDI position\": Value Change" {
      selector: _ -> [_ _ _ _ _ _ _ _ _ _ _ _]
      dyn-events: _ -> [_ _ _ _ _ _ _ _ _ _ _ _]
      timeout: 100 -> [_ _ _ _ _ _ _ _ _ _ _ _]
      tunnel: w56 -> [w72 w87 w109 w129 w276 w405 w439 w473 w507 w541 w575 w612]
      tunnel: [w72 w86 w109 w112 w260 w400 w434 w468 w502 w536 w570 w611] -> w55
      tunnel: w54 -> [w67 w81 w105 w125 w275 w422 w456 w490 w524 w558 w592 w610]
      tunnel: [w67 w81 w105 w125 w273 w422 w456 w490 w524 w558 w592 w610] -> w53
      tunnel: w52 -> [_ _ _ _ w269 _ _ _ _ _ _ _]
      tunnel: w51 -> [_ _ _ _ w268 _ _ _ _ _ _ w609]
      tunnel: [w71 w85 w91 w131 w267 w397 w432 w466 w499 w534 w568 w602] -> w50
      tunnel: w41 -> [w71 w85 w91 w131 _ w397 w432 w466 w499 w534 w568 w602]
      tunnel: [w70 w84 w108 w134 w266 w396 w431 w465 w498 w533 w567 w605] -> w49
      tunnel: w48 -> [w70 w84 w108 w134 w263 w396 w431 w465 w498 w533 w567 w605]
      tunnel: [w69 w83 w107 w133 w265 w399 w430 w467 w501 w532 w569 w604] -> w47
      tunnel: [w68 w82 w106 w132 w264 w398 w433 w464 w500 w535 w566 w603] -> w46
      tunnel: w45 -> [w69 w83 w107 w133 w262 w399 w430 w467 w501 w532 w569 w604]
      tunnel: w44 -> [w68 w82 w106 w132 w261 w398 w433 w464 w500 w535 w566 w603]
      tunnel: "how much sensors" -> [_ _ _ w130 w259 _ _ _ _ _ _ _]
      tunnel: w42 -> [_ _ _ _ w258 _ _ _ _ _ _ _]
      tunnel: w40 -> [w66 w80 w103 w135 w257 w423 w457 w491 w525 w559 w593 w601]
      tunnel: [w66 w80 w102 w135 w257 w423 w457 w491 w525 w559 w593 w601] -> w39
      tunnel: w38 -> [w65 w79 w101 w136 w256 w421 w455 w489 w523 w557 w591 w600]
      tunnel: [w65 w79 w99 w136 w256 w421 w455 w489 w523 w557 w591 w600] -> w37
      tunnel: 200.0 ("Speed") -> [_ _ _ _ _ w404 w438 w472 w506 w540 w574 _]
      tunnel: 10.0 ("Speed") -> [_ _ _ _ _ w403 w437 w471 w505 w539 w573 _]
      tunnel: w34 -> [_ _ _ w123 _ _ _ _ _ _ _ _]
      tunnel: w33 -> [_ _ _ w122 _ _ _ _ _ _ _ _]
      tunnel: w32 -> [_ _ _ w121 _ _ _ _ _ _ _ _]
      tunnel: [w61 w75 w94 w120 w252 w392 w426 w460 w494 w528 w562 w596] -> w31
      tunnel: w30 -> [w61 w75 w94 w119 w252 w392 w426 w460 w494 w528 w562 w596]
      tunnel: [w62 w76 w95 w118 w253 w393 w427 w461 w495 w529 w563 w597] -> w29
      tunnel: w28 -> [w62 w76 w95 w117 w253 w393 w427 w461 w495 w529 w563 w597]
      tunnel: [w63 w77 w96 w116 w254 w394 w428 w462 w496 w530 w564 w598] -> w27
      tunnel: w26 -> [w63 w77 w96 w115 w254 w394 w428 w462 w496 w530 w564 w598]
      tunnel: [w60 w74 w93 w114 w251 w391 w425 w459 w493 w527 w561 w595] -> w25
      tunnel: w24 -> [w60 w74 w93 _ w251 w391 w425 w459 w493 w527 w561 w595]
      tunnel: w22 -> [w64 w78 w98 w113 w255 w395 w429 w463 w497 w531 w565 w599]
      tunnel: [w64 w78 w97 w113 w255 w395 w429 w463 w497 w531 w565 w599] -> w23
      tunnel: [w59 w73 w89 w110 w250 w390 w424 w458 w492 w526 w560 w594] -> w20
      tunnel: w21 -> [w59 w73 w89 w111 w250 w390 w424 w458 w492 w526 w560 w594]
      event Timeout {
        n15 = event-data() -> ()  [unwired: 1 in, 3 out]
      }
      event "go to park": Value Change {
        n16 = event-data() -> ()  [unwired: 1 in, 6 out]
        n17 = call "XYZTheta Go.vi"("XYZTheta In"="Parking position", "Motion in"=w87) -> ("Motion out"=w86:refnum<class "Motion.lvclass">)  [unwired: 7 in, 2 out]
      }
      event "calculate": Value Change {
        n18 = event-data() -> ()  [unwired: 1 in, 6 out]
        n19 = Add(x=1.0, y=w103) -> (x+y=w102:dbl)
        n20 = Subtract(x=w93, y=dbl[][] [[0.4, 0.4, 0.0, 0.0], [0.4, 0.4, 0.0, 0.0]]) -> (x-y=w92:dbl[][])
        n21 = Subtract(x=w92, y=w91) -> (x-y=w100:dbl[][])
        "HDI - sensor deviation on time" <- w100
        n22 = Insert Into Array(array=w101, new element=w100) -> (w99:dbl[][][])  [unwired: 3 in]
        "HDI-sensor deviation from all time" <- w99
        n23 = Insert Into Array(array=w98, new element=w93) -> (w97:dbl[][][])  [unwired: 3 in]
        "HDI center position from all time" <- w97
        "HDI center position on time" <- w93
      }
      event "measure HDI position": Value Change {
        n24 = event-data() -> ()  [unwired: 1 in, 6 out]
        n25 = Add(x=1.0, y=w111) -> (x+y=w110:dbl)
        "measure times of HDI" <- w110
        n26 = Greater?(x=w110, y=1.0) -> (0:w126:bool)
        n27 = Not(x=w126) -> (.not. x?=w124:bool)
        n28 = case shown="False" w124 {
          tunnel: w129 -> [w138 w201]
          tunnel: [w139 w194] -> w112
          tunnel: w121 -> [_ w200]
          tunnel: w122 -> [_ w199]
          tunnel: [w143 w198] -> w114
          tunnel: [w146 w197] -> w116
          tunnel: [w145 w196] -> w118
          tunnel: [w144 w195] -> w120
          tunnel: w115 -> [w142 _]
          tunnel: w117 -> [w141 _]
          tunnel: w119 -> [w140 _]
          tunnel: w130 -> [w137 w193]
          tunnel: w123 -> [_ w192]
          frame False {
            n29 = for {
              N: w137 -> [_]
              shift-right: [w178] -> w139
              shift-left: w138 -> [w179]
              tunnel: [w169] -> w143 mode=indexing
              tunnel: [w174] -> w146 mode=indexing
              tunnel: [w173] -> w145 mode=indexing
              tunnel: [w172] -> w144 mode=indexing
              tunnel: w142 -> [w170] mode=indexing
              tunnel: w141 -> [w151] mode=indexing
              tunnel: w140 -> [w147] mode=indexing
              # "rotation"
              n30 = call "Joystick and Camera SHIH VPC- external Connection.vi"("Motion in"=w179, "XYZTheta"=w170, "Measurement Point"="Measure Top-Left  cross mark of HDI B", "Inital GO"=TRUE) -> ("Motion out"=w168:refnum<class "Motion.lvclass">, "Sum"=w174:dbl[])  [unwired: 3 in, 2 out]
              n31 = Array Subset(array=w151, index=0, length=2) -> (w152:dbl[])
              n32 = call-dynamic "XY Go.vi"("Speed"=100.0, "XY"=w152, "Motion in"=w168) -> ("Motion out"=w166:refnum<class "Motion.lvclass">)  [unwired: 7 in, 1 out]
              n33 = Index Array(array=w151, index=2) -> (element=w163:dbl)
              n34 = call-dynamic "Z Go.vi"("Speed"=10.0, "Position"=w163, "Motion in"=w166) -> ("Motion out"=w165:refnum<class "Motion.lvclass">)  [unwired: 7 in, 1 out]
              n35 = call "Joystick and Camera SHIH VPC- external Connection.vi"("Motion in"=w165, "Measurement Point"="Measure Bottom-Left cross mard of HDI B", "Inital GO"=FALSE) -> ("Motion out"=w158:refnum<class "Motion.lvclass">, "Sum"=w173:dbl[])  [unwired: 4 in, 2 out]
              n36 = Subtract(x=w173, y=w174) -> (x-y=w187:dbl[])
              n37 = Array Subset(array=w147, index=0, length=2) -> (w148:dbl[])
              n38 = call-dynamic "XY Go.vi"("Speed"=100.0, "XY"=w148, "Motion in"=w158) -> ("Motion out"=w160:refnum<class "Motion.lvclass">)  [unwired: 7 in, 1 out]
              n39 = Index Array(array=w147, index=2) -> (element=w155:dbl)
              n40 = call "XY_to_Rotation_RPHI.vi"("X-Y"=w187) -> ("r-phi"=w183:dbl[])
              n41 = call-dynamic "Z Go.vi"("Speed"=10.0, "Position"=w155, "Motion in"=w160) -> ("Motion out"=w157:refnum<class "Motion.lvclass">)  [unwired: 7 in, 1 out]
              n42 = Index Array(array=w183, index=1) -> (element=w180:dbl)
              n43 = call "Joystick and Camera SHIH VPC- external Connection.vi"("Motion in"=w157, "Measurement Point"="Measure Bottom-Righ cross mark of HDI B", "Inital GO"=FALSE) -> ("Motion out"=w178:refnum<class "Motion.lvclass">, "Sum"=w172:dbl[])  [unwired: 4 in, 2 out]
              n44 = Multiply(x=w180, y=-1.0) -> (x*y=w176:dbl)
              n45 = Add(x=w172, y=w174) -> (x+y=w190:dbl[])
              n46 = Divide(x=w190, y=2.0) -> (x/y=w175:dbl[])
              n47 = Replace Array Subset(array=w175, new element=w176, index=3) -> (w169:dbl[])
            }
          }
          frame True {
            n48 = for {
              N: w193 -> [_]
              tunnel: w200 -> [w218] mode=indexing
              shift-right: [w216] -> w194
              shift-left: w201 -> [w217]
              tunnel: w199 -> [w205]
              tunnel: [w202] -> w198 mode=indexing
              tunnel: [w212] -> w197 mode=indexing
              tunnel: [w211] -> w196 mode=indexing
              tunnel: [w210] -> w195 mode=indexing
              tunnel: w192 -> [w203]
              i -> [w207]
              # "rotation"
              n49 = Equal?(x=0, y=w207) -> (x = y?=w208:bool)
              n50 = case shown="False" w208 {
                tunnel: [w248 w249] -> w204
                tunnel: w205 -> [_ w249]
                tunnel: w203 -> [w248 _]
                frame False {
                }
                frame True {
                }
              }
              n51 = call "Joystick and Camera SHIH VPC- external Connection.vi"("Motion in"=w217, "XYZTheta"=w204, "Measurement Point"="Measure Top-Left  cross mark of HDI B", "Inital GO"=TRUE) -> ("Motion out"=w230:refnum<class "Motion.lvclass">, "Sum"=w212:dbl[])  [unwired: 3 in, 2 out]
              n52 = Add(x=w218, y=w212) -> (x+y=w234:dbl[])
              n53 = Index Array(array=w212, index=0) -> (element=w221:dbl)
              n54 = Array Subset(array=w234, index=0, length=2) -> (w233:dbl[])
              n55 = Replace Array Subset(array=w233, new element=w221, index=0) -> (w231:dbl[])
              n56 = call-dynamic "XY Go.vi"("Speed"=100.0, "XY"=w231, "Motion in"=w230) -> ("Motion out"=w238:refnum<class "Motion.lvclass">)  [unwired: 7 in, 1 out]
              n57 = call "Joystick and Camera SHIH VPC- external Connection.vi"("Motion in"=w238, "Measurement Point"="Measure Bottom-Left cross mard of HDI B", "Inital GO"=FALSE) -> ("Motion out"=w229:refnum<class "Motion.lvclass">, "Sum"=w211:dbl[])  [unwired: 4 in, 2 out]
              n58 = Array Subset(array=w234, index=0, length=2) -> (w240:dbl[])
              n59 = Subtract(x=w211, y=w212) -> (x-y=w228:dbl[])
              n60 = call-dynamic "XY Go.vi"("Speed"=100.0, "XY"=w240, "Motion in"=w229) -> ("Motion out"=w244:refnum<class "Motion.lvclass">)  [unwired: 7 in, 1 out]
              n61 = call "XY_to_Rotation_RPHI.vi"("X-Y"=w228) -> ("r-phi"=w224:dbl[])
              n62 = call "Joystick and Camera SHIH VPC- external Connection.vi"("Motion in"=w244, "Measurement Point"="Measure Bottom-Righ cross mark of HDI B", "Inital GO"=FALSE) -> ("Motion out"=w216:refnum<class "Motion.lvclass">, "Sum"=w210:dbl[])  [unwired: 4 in, 2 out]
              n63 = Index Array(array=w224, index=1) -> (element=w219:dbl)
              n64 = Multiply(x=w219, y=-1.0) -> (x*y=w214:dbl)
              n65 = Add(x=w210, y=w212) -> (x+y=w246:dbl[])
              n66 = Divide(x=w246, y=2.0) -> (x/y=w213:dbl[])
              n67 = Replace Array Subset(array=w213, new element=w214, index=3) -> (w202:dbl[])
            }
          }
        }
      }
      event "measure sensor position": Value Change {
        n68 = event-data() -> ()  [unwired: 1 in, 6 out]
        n69 = Add(x=1.0, y=w275) -> (x+y=w273:dbl)
        "measure times of sensor" <- w273
        n70 = Greater?(x=w273, y=1.0) -> (0:w271:bool)
        n71 = Not(x=w271) -> (.not. x?=w270:bool)
        n72 = case shown="True" w270 {
          tunnel: w276 -> [w278 w341]
          tunnel: [w279 w334] -> w260
          tunnel: w269 -> [_ w340]
          tunnel: w268 -> [_ w339]
          tunnel: [w283 w338] -> w267
          tunnel: [w286 w337] -> w266
          tunnel: [w285 w336] -> w265
          tunnel: [w284 w335] -> w264
          tunnel: w263 -> [w282 _]
          tunnel: w262 -> [w281 _]
          tunnel: w261 -> [w280 _]
          tunnel: w259 -> [w277 w333]
          tunnel: w258 -> [_ w332]
          frame False {
            n73 = for {
              N: w277 -> [_]
              shift-right: [w318] -> w279
              shift-left: w278 -> [w319]
              tunnel: [w309] -> w283 mode=indexing
              tunnel: [w314] -> w286 mode=indexing
              tunnel: [w313] -> w285 mode=indexing
              tunnel: [w312] -> w284 mode=indexing
              tunnel: w282 -> [w310] mode=indexing
              tunnel: w281 -> [w292] mode=indexing
              tunnel: w280 -> [w288] mode=indexing
              # "rotation"
              n74 = call "Joystick and Camera SHIH VPC- external Connection.vi"("Motion in"=w319, "XYZTheta"=w310, "Measurement Point"="Measure Top-Left  cross mark of sensor B", "Inital GO"=TRUE) -> ("Motion out"=w304:refnum<class "Motion.lvclass">, "Sum"=w314:dbl[])  [unwired: 3 in, 2 out]
              n75 = Array Subset(array=w292, index=0, length=2) -> (w291:dbl[])
              n76 = call-dynamic "XY Go.vi"("Speed"=100.0, "XY"=w291, "Motion in"=w304) -> ("Motion out"=w306:refnum<class "Motion.lvclass">)  [unwired: 7 in, 1 out]
              n77 = Index Array(array=w292, index=2) -> (element=w302:dbl)
              n78 = call-dynamic "Z Go.vi"("Speed"=10.0, "Position"=w302, "Motion in"=w306) -> ("Motion out"=w303:refnum<class "Motion.lvclass">)  [unwired: 7 in, 1 out]
              n79 = call "Joystick and Camera SHIH VPC- external Connection.vi"("Motion in"=w303, "Measurement Point"="Measure Bottom-Left cross mard of sensor B", "Inital GO"=FALSE) -> ("Motion out"=w298:refnum<class "Motion.lvclass">, "Sum"=w313:dbl[])  [unwired: 4 in, 2 out]
              n80 = Subtract(x=w313, y=w314) -> (x-y=w327:dbl[])
              n81 = Array Subset(array=w288, index=0, length=2) -> (w287:dbl[])
              n82 = call-dynamic "XY Go.vi"("Speed"=100.0, "XY"=w287, "Motion in"=w298) -> ("Motion out"=w300:refnum<class "Motion.lvclass">)  [unwired: 7 in, 1 out]
              n83 = Index Array(array=w288, index=2) -> (element=w295:dbl)
              n84 = call "XY_to_Rotation_RPHI.vi"("X-Y"=w327) -> ("r-phi"=w323:dbl[])
              n85 = call-dynamic "Z Go.vi"("Speed"=10.0, "Position"=w295, "Motion in"=w300) -> ("Motion out"=w297:refnum<class "Motion.lvclass">)  [unwired: 7 in, 1 out]
              n86 = Index Array(array=w323, index=1) -> (element=w320:dbl)
              n87 = Multiply(x=w320, y=-1.0) -> (x*y=w316:dbl)
              n88 = call "Joystick and Camera SHIH VPC- external Connection.vi"("Motion in"=w297, "Measurement Point"="Measure Bottom-Righ cross mark of sensor B", "Inital GO"=FALSE) -> ("Motion out"=w318:refnum<class "Motion.lvclass">, "Sum"=w312:dbl[])  [unwired: 4 in, 2 out]
              n89 = Add(x=w312, y=w314) -> (x+y=w330:dbl[])
              n90 = Divide(x=w330, y=2.0) -> (x/y=w315:dbl[])
              n91 = Replace Array Subset(array=w315, new element=w316, index=3) -> (w309:dbl[])
            }
          }
          frame True {
            n92 = for {
              N: w333 -> [_]
              tunnel: w340 -> [w358] mode=indexing
              shift-right: [w356] -> w334
              shift-left: w341 -> [w357]
              tunnel: w339 -> [w345]
              tunnel: [w342] -> w338 mode=indexing
              tunnel: [w352] -> w337 mode=indexing
              tunnel: [w351] -> w336 mode=indexing
              tunnel: [w350] -> w335 mode=indexing
              tunnel: w332 -> [w343]
              i -> [w347]
              # "rotation"
              n93 = Equal?(x=0, y=w347) -> (x = y?=w348:bool)
              n94 = case shown="True" w348 {
                tunnel: [w388 w389] -> w344
                tunnel: w345 -> [_ w389]
                tunnel: w343 -> [w388 _]
                frame False {
                }
                frame True {
                }
              }
              n95 = call "Joystick and Camera SHIH VPC- external Connection.vi"("Motion in"=w357, "XYZTheta"=w344, "Measurement Point"="Measure Top-Left  cross mark of sensor B", "Inital GO"=TRUE) -> ("Motion out"=w370:refnum<class "Motion.lvclass">, "Sum"=w352:dbl[])  [unwired: 3 in, 2 out]
              n96 = Add(x=w358, y=w352) -> (x+y=w374:dbl[])
              n97 = Index Array(array=w352, index=0) -> (element=w361:dbl)
              n98 = Array Subset(array=w374, index=0, length=2) -> (w373:dbl[])
              n99 = Replace Array Subset(array=w373, new element=w361, index=0) -> (w371:dbl[])
              n100 = call-dynamic "XY Go.vi"("Speed"=100.0, "XY"=w371, "Motion in"=w370) -> ("Motion out"=w378:refnum<class "Motion.lvclass">)  [unwired: 7 in, 1 out]
              n101 = call "Joystick and Camera SHIH VPC- external Connection.vi"("Motion in"=w378, "Measurement Point"="Measure Bottom-Left cross mard of sensor B", "Inital GO"=FALSE) -> ("Motion out"=w369:refnum<class "Motion.lvclass">, "Sum"=w351:dbl[])  [unwired: 4 in, 2 out]
              n102 = Array Subset(array=w374, index=0, length=2) -> (w380:dbl[])
              n103 = Subtract(x=w351, y=w352) -> (x-y=w368:dbl[])
              n104 = call-dynamic "XY Go.vi"("Speed"=100.0, "XY"=w380, "Motion in"=w369) -> ("Motion out"=w384:refnum<class "Motion.lvclass">)  [unwired: 7 in, 1 out]
              n105 = call "XY_to_Rotation_RPHI.vi"("X-Y"=w368) -> ("r-phi"=w364:dbl[])
              n106 = call "Joystick and Camera SHIH VPC- external Connection.vi"("Motion in"=w384, "Measurement Point"="Measure Bottom-Righ cross mark of sensor B", "Inital GO"=FALSE) -> ("Motion out"=w356:refnum<class "Motion.lvclass">, "Sum"=w350:dbl[])  [unwired: 4 in, 2 out]
              n107 = Index Array(array=w364, index=1) -> (element=w359:dbl)
              n108 = Multiply(x=w359, y=-1.0) -> (x*y=w354:dbl)
              n109 = Add(x=w350, y=w352) -> (x+y=w386:dbl[])
              n110 = Divide(x=w386, y=2.0) -> (x/y=w353:dbl[])
              n111 = Replace Array Subset(array=w353, new element=w354, index=3) -> (w342:dbl[])
            }
          }
        }
      }
      event "north - upper left": Value Change {
        n112 = event-data() -> ()  [unwired: 1 in, 6 out]
        n113 = Array Subset(array=w396, index (row)=0 ("index"), length (row)=1 ("length"), index (col)=0 ("index"), length (col)=4 ("length")) -> (w416:dbl[][])
        n114 = Reshape Array(w416, 4 ("dimension size")) -> (w414:dbl[])
        n115 = Index Array(array=w414, index #1=0 ("index"), index #2=1 ("index"), index #3=2 ("index")) -> (element #1=w410:dbl, element #2=w409:dbl, element #3=w407:dbl)
        n116 = Build Array(w410, w409) -> (w408:dbl[])
        n117 = call-dynamic "XY Go.vi"("Speed"=w404, "XY"=w408, "Motion in"=w405) -> ("Motion out"=w406:refnum<class "Motion.lvclass">)  [unwired: 7 in, 1 out]
        n118 = call-dynamic "Z Go.vi"("Speed"=w403, "Position"=w407, "Motion in"=w406) -> ("Motion out"=w402:refnum<class "Motion.lvclass">)  [unwired: 7 in, 1 out]
        n119 = call "Joystick and Camera SHIH VPC- external Connection.vi"("Motion in"=w402, "Inital GO"=FALSE) -> ("Motion out"=w400:refnum<class "Motion.lvclass">)  [unwired: 5 in, 3 out]
      }
      event "north - bottom left": Value Change {
        n120 = event-data() -> ()  [unwired: 1 in, 6 out]
        n121 = Array Subset(array=w430, index (row)=0 ("index"), length (row)=1 ("length"), index (col)=0 ("index"), length (col)=4 ("length")) -> (w450:dbl[][])
        n122 = Reshape Array(w450, 4 ("dimension size")) -> (w448:dbl[])
        n123 = Index Array(array=w448, index #1=0 ("index"), index #2=1 ("index"), index #3=2 ("index")) -> (element #1=w444:dbl, element #2=w443:dbl, element #3=w441:dbl)
        n124 = Build Array(w444, w443) -> (w442:dbl[])
        n125 = call-dynamic "XY Go.vi"("Speed"=w438, "XY"=w442, "Motion in"=w439) -> ("Motion out"=w440:refnum<class "Motion.lvclass">)  [unwired: 7 in, 1 out]
        n126 = call-dynamic "Z Go.vi"("Speed"=w437, "Position"=w441, "Motion in"=w440) -> ("Motion out"=w436:refnum<class "Motion.lvclass">)  [unwired: 7 in, 1 out]
        n127 = call "Joystick and Camera SHIH VPC- external Connection.vi"("Motion in"=w436, "Inital GO"=FALSE) -> ("Motion out"=w434:refnum<class "Motion.lvclass">)  [unwired: 5 in, 3 out]
      }
      event "north - bottom right": Value Change {
        n128 = event-data() -> ()  [unwired: 1 in, 6 out]
        n129 = Array Subset(array=w464, index (row)=0 ("index"), length (row)=1 ("length"), index (col)=0 ("index"), length (col)=4 ("length")) -> (w484:dbl[][])
        n130 = Reshape Array(w484, 4 ("dimension size")) -> (w482:dbl[])
        n131 = Index Array(array=w482, index #1=0 ("index"), index #2=1 ("index"), index #3=2 ("index")) -> (element #1=w478:dbl, element #2=w477:dbl, element #3=w475:dbl)
        n132 = Build Array(w478, w477) -> (w476:dbl[])
        n133 = call-dynamic "XY Go.vi"("Speed"=w472, "XY"=w476, "Motion in"=w473) -> ("Motion out"=w474:refnum<class "Motion.lvclass">)  [unwired: 7 in, 1 out]
        n134 = call-dynamic "Z Go.vi"("Speed"=w471, "Position"=w475, "Motion in"=w474) -> ("Motion out"=w470:refnum<class "Motion.lvclass">)  [unwired: 7 in, 1 out]
        n135 = call "Joystick and Camera SHIH VPC- external Connection.vi"("Motion in"=w470, "Inital GO"=FALSE) -> ("Motion out"=w468:refnum<class "Motion.lvclass">)  [unwired: 5 in, 3 out]
      }
      event "south - upper left": Value Change {
        n136 = event-data() -> ()  [unwired: 1 in, 6 out]
        n137 = Array Subset(array=w498, index (row)=1 ("index"), length (row)=1 ("length"), index (col)=0 ("index"), length (col)=4 ("length")) -> (w518:dbl[][])
        n138 = Reshape Array(w518, 4 ("dimension size")) -> (w516:dbl[])
        n139 = Index Array(array=w516, index #1=0 ("index"), index #2=1 ("index"), index #3=2 ("index")) -> (element #1=w512:dbl, element #2=w511:dbl, element #3=w509:dbl)
        n140 = Build Array(w512, w511) -> (w510:dbl[])
        n141 = call-dynamic "XY Go.vi"("Speed"=w506, "XY"=w510, "Motion in"=w507) -> ("Motion out"=w508:refnum<class "Motion.lvclass">)  [unwired: 7 in, 1 out]
        n142 = call-dynamic "Z Go.vi"("Speed"=w505, "Position"=w509, "Motion in"=w508) -> ("Motion out"=w504:refnum<class "Motion.lvclass">)  [unwired: 7 in, 1 out]
        n143 = call "Joystick and Camera SHIH VPC- external Connection.vi"("Motion in"=w504, "Inital GO"=FALSE) -> ("Motion out"=w502:refnum<class "Motion.lvclass">)  [unwired: 5 in, 3 out]
      }
      event "south - bottom left": Value Change {
        n144 = event-data() -> ()  [unwired: 1 in, 6 out]
        n145 = Array Subset(array=w532, index (row)=1 ("index"), length (row)=1 ("length"), index (col)=0 ("index"), length (col)=4 ("length")) -> (w552:dbl[][])
        n146 = Reshape Array(w552, 4 ("dimension size")) -> (w550:dbl[])
        n147 = Index Array(array=w550, index #1=0 ("index"), index #2=1 ("index"), index #3=2 ("index")) -> (element #1=w546:dbl, element #2=w545:dbl, element #3=w543:dbl)
        n148 = Build Array(w546, w545) -> (w544:dbl[])
        n149 = call-dynamic "XY Go.vi"("Speed"=w540, "XY"=w544, "Motion in"=w541) -> ("Motion out"=w542:refnum<class "Motion.lvclass">)  [unwired: 7 in, 1 out]
        n150 = call-dynamic "Z Go.vi"("Speed"=w539, "Position"=w543, "Motion in"=w542) -> ("Motion out"=w538:refnum<class "Motion.lvclass">)  [unwired: 7 in, 1 out]
        n151 = call "Joystick and Camera SHIH VPC- external Connection.vi"("Motion in"=w538, "Inital GO"=FALSE) -> ("Motion out"=w536:refnum<class "Motion.lvclass">)  [unwired: 5 in, 3 out]
      }
      event "south - bottom right": Value Change {
        n152 = event-data() -> ()  [unwired: 1 in, 6 out]
        n153 = Array Subset(array=w566, index (row)=1 ("index"), length (row)=1 ("length"), index (col)=0 ("index"), length (col)=4 ("length")) -> (w586:dbl[][])
        n154 = Reshape Array(w586, 4 ("dimension size")) -> (w584:dbl[])
        n155 = Index Array(array=w584, index #1=0 ("index"), index #2=1 ("index"), index #3=2 ("index")) -> (element #1=w580:dbl, element #2=w579:dbl, element #3=w577:dbl)
        n156 = Build Array(w580, w579) -> (w578:dbl[])
        n157 = call-dynamic "XY Go.vi"("Speed"=w574, "XY"=w578, "Motion in"=w575) -> ("Motion out"=w576:refnum<class "Motion.lvclass">)  [unwired: 7 in, 1 out]
        n158 = call-dynamic "Z Go.vi"("Speed"=w573, "Position"=w577, "Motion in"=w576) -> ("Motion out"=w572:refnum<class "Motion.lvclass">)  [unwired: 7 in, 1 out]
        n159 = call "Joystick and Camera SHIH VPC- external Connection.vi"("Motion in"=w572, "Inital GO"=FALSE) -> ("Motion out"=w570:refnum<class "Motion.lvclass">)  [unwired: 5 in, 3 out]
      }
      event "test": Value Change {
        n160 = event-data() -> ()  [unwired: 1 in, 6 out]
        n161 = Equal?(x=0.0, y=0.0) -> (x = y?=w606:bool)
        n162 = case shown="True" w606 {
          tunnel: w612 -> [w613 w617]
          tunnel: [w613 w616] -> w611
          tunnel: w609 -> [_ w615]
          frame False {
          }
          frame True {
            n163 = for {
              N: 2 -> [_]
              tunnel: w615 -> [w619]
              shift-right: [w620] -> w616
              shift-left: w617 -> [w621]
              n164 = call "Joystick and Camera SHIH VPC- external Connection.vi"("Motion in"=w621, "XYZTheta"=w619, "Inital GO"=TRUE) -> ("Motion out"=w620:refnum<class "Motion.lvclass">)  [unwired: 4 in, 3 out]
            }
          }
        }
      }
    }
    n165 = feedback-in #1(w27) -> ()
    n166 = feedback-in #2(w49) -> ()
    n167 = feedback-in #3(w29) -> ()
    n168 = feedback-in #4(w47) -> ()
    n169 = feedback-in #5(w46) -> ()
    n170 = feedback-in #6(w31) -> ()
    n171 = feedback-in #7(w50) -> ()
    n172 = feedback-in #8(w25) -> ()
  }
  n173 = call-dynamic "Disconnect.vi"("Controller in"=w16) -> ()  [unwired: 9 in, 1 out]
